vi "UNITEST MAIN.vi"() -> ()   [LabVIEW 2025]
uses:
  controls/LAB-IQ UI Data.ctl
  support/Message Queue/Enqueue Message (Single).vi
  <vilib>/Utility/error.llb/Error Cluster From Error Code.vi
  <vilib>/ErrorRing/Error Ring.xnode
  support/Message Queue/LAB-IQ Message Queue.lvlib
  support/User Event - Stop/LAB-IQ User Event - Stop.lvlib
panel:
  in  "Tab Control 3":T1(tab)
  in  "Tab Control 5":enum32{""}(tab)
  in  "Tab Control 14":T2(tab)=enum."Motor Load"
  out "sample temp":dbl caption="Sample Temperature" min=-200.0 max=200.0 step=0.1 format="%.1f"
  in  "output range":cluster{"output high":dbl, "output low":dbl}={"output high"=80.0, "output low"=0.0} {"output low" format="%.2f"; "output high" format="%.2f"}
  in  "PID gains out":T3={"proportional gain (Kc)"=40.0, "integral time (Ti, min)"=0.09, "derivative time (Td, min)"=0.0} {"derivative time (Td, min)" format="%.3f"; "integral time (Ti, min)" format="%.3f"; "proportional gain (Kc)" format="%.3f"}
  out "HT PID o/p":dbl
  in  "reinit":bool=TRUE
  out "gFF Rot 6":cluster{dbl, dbl, dbl}(graph)
  out "HT PID o/p 2":dbl
  in  "reinit 2":bool=TRUE
  in  "PID gains out 2":T3={"proportional gain (Kc)"=10.0, "integral time (Ti, min)"=1.667, "derivative time (Td, min)"=0.0} {"derivative time (Td, min)" format="%.3f"; "integral time (Ti, min)" format="%.3f"; "proportional gain (Kc)" format="%.3f"}
  in  "output range 3":cluster{"output high":dbl, "output low":dbl}={"output high"=80.0, "output low"=0.0} {"output low" format="%.2f"; "output high" format="%.2f"}
  out "gFF Rot 8":cluster{dbl, dbl, dbl}(graph)
  in  "Ramp MulFac":dbl=2.0
  in  "pulses LoadDiffRamp(2..10)":dbl=9.0
  in  "PulseControlRamp(diff<=3N)":dbl=5.0 min=1.0 max=1000.0 step=1.0 format="%#.1f"
  in  "SetLoadDeadband(%) Load(0-10N)":dbl=0.1 min=0.0001 max=100.0 step=0.0001 format="%#.6f"
  in  "PID gains out delay (microForce)":T3={"proportional gain (Kc)"=300.0, "integral time (Ti, min)"=0.00011, "derivative time (Td, min)"=0.0} {"derivative time (Td, min)" format="%.3f"; "integral time (Ti, min)" min=1e-05 max=100.0 step=1e-06 format="%.6f"; "proportional gain (Kc)" format="%.3f"}
  in  "Ramp":bool
  in  "Gain 2":dbl=0.016
  in  "pulses LoadDiff(2..10)":dbl=10.0
  in  "pulses LoadDiff(11..50)":dbl=40.0
  in  "PulseControl(diff<=3N)":dbl=1.0 min=1.0 max=1000.0 step=1.0 format="%#.1f"
  out "SetLoadDeadband(%)  2":dbl=1.0 min=0.001 max=100.0 step=0.001 format="%#.6f"
  in  "Dummy Run":bool
  out "Vertical load (N)":dbl format="%#.3f"
  in  "AutoTune":bool
  in  "Offset  3":dbl=1.5
  in  "apply load":bool
  in  "Enter ByPass Load":dbl
  in  "reinit 3":bool=TRUE
  in  "output range delay":cluster{"output high":dbl, "output low":dbl}={"output high"=100.0, "output low"=-100.0} {"output low" format="%.2f"; "output high" format="%.2f"}
  in  "PID gains out delay":T3={"proportional gain (Kc)"=30.0, "integral time (Ti, min)"=0.00101, "derivative time (Td, min)"=0.0} {"derivative time (Td, min)" format="%.3f"; "integral time (Ti, min)" min=1e-05 max=100.0 step=0.0001 format="%.4f"; "proportional gain (Kc)" format="%.3f"}
  in  "Bypass Load":bool
  in  "pulsesSent":dbl=200.0
  out "pulses":dbl
  out "actpid":dbl
  out "gFF Rot 7":cluster{dbl, dbl, dbl}(graph)
  in  "pulses LoadDiff(21..1000)":dbl=40.0
  in  "Delay":dbl=1.5 min=0.001 max=5.0 step=0.001 format="%#.6f"
  in  "deadband":dbl=0.2
  in  "Tab Control 26":enum32{"Page 1", "Page 2"}(tab)
  in  "ClearAll":bool
  out "Mz(Nm)":dbl[](array[numeric])
  out "My(Nm)":dbl[](array[numeric])
  out "Mx(Nm)":dbl[](array[numeric])
  in  "Save Dwell":dbl=0.015 caption="Save Dwell (sec)" min=0.0 max=5.0 step=0.001 format="%.3f"
  out "Set Speed 2":dbl
  out "Mx":dbl[](graph)
  out "My":dbl[](graph)
  out "Mz":dbl[](graph)
  out "Fx(N)":dbl[](graph)
  out "Fy(N)":dbl[](graph)
  out "Fz(N)":dbl[](graph)
  in  "ZeroAll":bool
  in  "Acq Delay (ms)":dbl=10.0
  in  "Burst Delay (ms)":dbl=10.0
  out "model":string
  out "SN":i32
  out "FFx(N)":dbl[](array[numeric])
  in  "Sensor IP":string="192.168.1.100"
  in  "Port":i32=8080
  out "FFy(N)":dbl[](array[numeric])
  out "Load(N)":dbl[](array[numeric])
  out "AE":bool
  in  "delete Handle":bool
  in  "Create Handle":bool=TRUE
  out "ft_data":dbl[](array[numeric])=[1.0, 1.0, 1.0, 1.0, 1.0, 1.0]
  out "ft_range":dbl[](array[numeric])=[1.0, 1.0, 1.0, 1.0, 1.0, 1.0]
  in  "stop 6":bool
  out "running_flag":bool
  out "ft_udp_handle":i32
  out "get-data-return":i32
  out "get-range-return":i32
  out "zero-return":i32
  out "filter-return":i32
  out "initial-return":i32
  out "deleteHandle-result":i32
  out "NL Kg":dbl caption="Normal Kg" min=-2000.0 max=2000.0 step=1.0 format="%.2f"
  in  "zFF 4":bool
  in  "APPLY":bool
  in  "Bypass":bool caption="Bypass to Manual load"
  in  "SP":dbl caption="SV ( N )" min=0.0 max=550.0 step=0.1 format="%.1f"
  in  "EGUpM":dbl=1500.0
  in  "Bypass 3":bool caption="Bypass  PID"
  in  "Control voltage":dbl caption="Control Voltage" min=0.0 max=10.0 step=0.01 format="%#.3f"
  out "NL":dbl caption="Normal Load ( N )" min=-2000.0 max=2000.0 step=1.0 format="%.2f"
  in  "Load 3":bool
  in  "Timer":dbl=1.0 min=0.0 max=50.0 step=1.0 format="%#.0f"
  out "Slide":dbl(slide) min=0.0 max=5.0 step=0.0001 scale=0.0..9.18
  in  "Approach \nVoltage":dbl min=0.0 max=2.0 step=0.01 format="%.2f"
  in  "PID gains < 10":T3={"proportional gain (Kc)"=0.032999999999999995, "integral time (Ti, min)"=0.019000000000000003, "derivative time (Td, min)"=0.0}
  in  "output range 2":cluster{"output high":dbl, "output low":dbl}={"output high"=9.18, "output low"=0.0}
  out "Chart 9":T4(graph)
  out "step size":i32=1
  out "Set Time":dbl
  out "Load 2":dbl
  out "Step Timer":dbl format="%<%H:%M:%S>t"
  in  "Sequence Counter":dbl
  in  "No of Sequence":i32 min=0 max=450 step=1
  in  "Depth gain R":dbl=0.5
  in  "Depth gain L":dbl=0.005
  out "Depth 2":cluster{dbl, dbl}(graph)
  out "HT PID output 2":dbl(slide) scale=0.0..100.0
  in  "zFF 5":bool
  out "FrictionKg":dbl caption="Friction Kg" min=-2000.0 max=2000.0 step=1.0 format="%.2f"
  out "friction":dbl caption="friction N" min=-2000.0 max=2000.0 step=1.0 format="%.2f"
  out "XY Graph 23":cluster{"scratch array-x":dbl[], dbl[]}(graph)
  out "XY Graph 24":cluster{"scratch array-x":dbl[], dbl[]}(graph)
  out "XY Graph 14":cluster{"scratch array-x":dbl[], dbl[]}(graph)
  out "XY Graph 13":cluster{"scratch array-x":dbl[], dbl[]}(graph)
  out "XY Graph 12":cluster{"scratch array-x":dbl[], dbl[]}(graph)
  in  "Tab Control 19":enum32{"Platform COM", "Config ", "DevInfo"}(tab)=enum."Config "
  in  "SAMPLES":dbl=100.0
  in  "Re-initilaize":bool
  in  "Filter ON/OFF":bool=TRUE
  in  "TracHomeSurgeOffsetCounts 10MM":dbl=505100.0
  in  "TracHomeSwayOffsetCounts 10MM":dbl=1432.0
  in  "Acoustic Emission:":dbl=1.0 min=0.0001 max=200.0 step=0.0001 format="%.4f"
  in  "Apply Filter (FF)":bool
  in  "Filter% 2":dbl=50.0 min=50.0 max=100.0 step=0.1 format="%.1f"
  in  "Apply Filter (Load)":bool=TRUE
  in  "Filter%":dbl=80.0 min=50.0 max=100.0 step=0.1 format="%.1f"
  in  "Sway distance (mm)":dbl=245.0
  in  "Surge distance (mm)":dbl=370.0
  in  "DataSavingLoopDelay(ms)":dbl=15.0
  in  "SAVE  2":bool
  in  "Enter Distance":bool caption="Enter Counts"
  in  "Sway Counts:":dbl=100.0 min=0.0 max=100000000.0 step=1.0 format="%.2f"
  in  "Distance (mm): 3":dbl=100.0 caption="Distance (mm):" min=0.0 max=1500.0 step=0.001 format="%.5f"
  in  "Surge Counts:":dbl=100.0 min=0.0 max=100000000.0 step=1.0 format="%.1f"
  in  "Distance (mm): 2":dbl=100.0 caption="Distance (mm):" min=0.0 max=1500.0 step=0.0001 format="%.3f"
  in  "Distance (mm):":dbl=100.0 min=0.0 max=1500.0 step=0.001 format="%.5f"
  in  "Heave Counts:":dbl=100.0 min=0.0 max=100000000.0 step=1.0
  in  "LRMHomeSurgeOffsetCounts":dbl=307197.0
  in  "LRMHomeSwayOffsetCounts":dbl=26880.0
  in  "TracHomeSurgeOffsetCounts 20MM":dbl=505100.0
  in  "TracHomeSwayOffsetCounts 20MM":dbl=1432.0
  in  "RotHomeSwayOffsetCounts":dbl=14656.0
  in  "RotHomeSurgeOffsetCounts":dbl=311465.0
  in  "Heave distance":dbl=340.0
  out "Zmm":dbl=1600.0
  out "Heave Pulses/mm":dbl=1600.0
  out "Surge Pulses/mm":dbl=1600.0
  out "Sway Pulses/mm":dbl=320.0
  in  "Heave Pitch":dbl=4.0
  in  "Surge Pitch":dbl=3.0
  in  "Sway Pitch":dbl=2.0
  in  "Heave PPR":dbl=6400.0
  in  "Surge PPR":dbl=6400.0
  in  "Sway PPR":dbl=6400.0
  in  "Step Speed":enum32{"Step Speed", "Step (load-Speed)"}(tab)
  in  "StepTable For Speed":string[][](table)=[["", "", ""], ["", "", ""], ["", "", ""], ["", "", ""]]
  in  "StepTable For Load-Speed":string[][](table)=[["", "", ""], ["", "", ""], ["", "", ""], ["", "", ""]]
  in  "GUI":T5(tab)
  in  "Platform Settings":bool caption="Password"
  in  "Configure":bool caption="Password"
  in  "Home":bool caption="Password"
  in  "EXIT":bool
  in  "Analysis":bool caption="Password"
  in  "service 2":bool caption="Password"
  in  "MainPage":T6(tab)=enum."HOME"
  in  "Select Load Head":bool
  in  "Notes :":string
  in  "FILE":string
  in  "Sample ID :":string
  in  "Operator ID :":string
  in  "Operator Name :":string
  in  "Auto":bool caption="Power Status"
  out "mm/s  Surge":dbl=7.0 caption="Jog" min=0.001 max=50.0 step=0.0001 format="%.2f"
  in  "Update Surge Speed":bool
  out "Drive Error":string
  in  "Disable Axis Jog Soft Limits":bool
  out "mm/s  Sway":dbl=7.0 caption="Jog" min=0.001 max=50.0 step=0.0001 format="%.2f"
  out "Sway and Surge COM Status":bool=TRUE caption="Load COM Status"
  out "Heave COM Status":bool=TRUE caption="Load COM Status"
  in  "Enable Platform":bool
  in  "Surge Forward Main":bool
  in  "Surge Backward Main":bool
  in  "Sway Right Main":bool
  in  "Sway Left Main":bool
  in  "Heave Down Main":bool
  in  "Heave Up main":bool
  in  "Update Sway Speed":bool
  in  "Update Heave Speed":bool
  out "mm/s Heave":dbl=7.0 caption="Jog" min=0.001 max=30.0 step=0.0001 format="%.2f"
  in  "mm/sec":dbl=1.0 caption="Jog" min=0.001 max=50.0 step=0.001 format="%.2f"
  in  "mm":dbl=0.001 caption="Jog" min=0.001 max=200.0 step=0.0001 format="%#.3f"
  in  "Surface Analysis":bool
  in  "Imaging":bool
  in  "Image Analysis":bool
  in  "Post Analysis":bool
  in  "Enter the Loading Rate (N/min)":dbl=60.0 min=60.0 max=1200.0 step=0.1 format="%.2f"
  out "Message":string="Load Entered is out of range!!!"
  out "Warning 2":bool
  in  "SSP 0.75":bool
  in  "SSP 0.5":bool
  in  "SSP 0.3":bool
  in  "Warning":enum32{"Page 2"}(tab)
  in  "gui GIF":enum32{"Check", "Deca", "kilo", "Micro"}(tab)
  out "Communication is established":bool=TRUE caption="Load COM Status"
  in  "AppLoad 4":bool
  in  "Multipoint":bool caption="Singlepoint"
  in  "Indentation":string[][](table)=[["Detection", "5", "2"], ["Unload", "0", "5"], ["Load", "10", "2"], ["Unload", "0", "5"], ["Detection", "5", "2"], ["Unload", "0", "5"]]
  in  "Reference Sample":u16(ring) items=["None", "Brass", "Aluminium", "Mild Steel"]
  out "Load Cell Communication Slide":u8(slide)=1 min=1 max=10 step=1 scale=0.0..10.0
  in  "com 3":bool
  out "com":bool
  out "DecaForce COM Status":bool caption="Load COM Status"
  in  "Update":bool
  in  "Clear 3":bool
  in  "seq":bool=TRUE
  in  "Stribeck table":bool
  in  "Stribeck Table  For loading":string[][](table)=[["", "", ""], ["", "", ""], ["", "", ""], ["", "", ""]]
  in  "Loading Mode":u16(ring) items=["Constant", "Ramp", "Steps", "Indentation"]
  in  "Enter the Final Load (N)":dbl=1.0 min=0.0 max=500.0 step=1.0 format="%#.0f"
  in  "Enter the CoF Trip":dbl=1.0
  in  "Enter the Friction Force Trip":dbl=520.0 min=500.0 max=500.0 step=1.0 format="%#.1f"
  in  "Enter the Normal load Trip":dbl=520.0 min=500.0 max=500.0 step=0.001 format="%.3f"
  in  "Enter the Load  (N)":dbl=2.0 min=0.0 max=500.0 step=0.1 format="%#.4f"
  in  "KiloForce":bool
  in  "DecaForce":bool
  in  "MicroForce":bool
  in  "LHBack":bool
  in  "LHNext":bool
  in  "zNL":bool
  out "NL disp":dbl caption="Normal Load ( N )" min=-2000.0 max=2000.0 step=0.0001 format="%.1f"
  in  "Rotary Tab":enum32{"Page 1", "Page 2"}(tab)
  in  "Motion Direction:  3":u16(ring) items=["Clockwise", "Counter Clockwise"]
  in  "E.Velocity 2":bool=TRUE caption="SRR"
  out "e.v/ssr 2":enum32{"E.V", "SSR"}(tab)
  in  "Enter Fixed SRR 2":dbl min=0.0 max=0.0 format="%.3f"
  in  "Enter the Final E.Velocity (m/s) 2":dbl=1.0 min=0.001 max=4.0 step=0.001 format="%.3f"
  in  "Enter initial E.Velocity (m/s) 2":dbl=2.0 min=0.001 max=4.0 step=0.001 format="%.3f"
  in  "Enter Fixed E.Velocity 2":dbl=1.0 min=0.001 max=2.0 step=0.001 format="%.3f"
  in  "Enter Final SRR 2":dbl=1.0 min=0.001 max=1.0 step=0.001 format="%.2f"
  in  "Enter initial SRR 2":dbl=1.0 min=0.001 max=1.0 step=0.001 format="%.2f"
  out "Final Speed (RPM) 3":dbl=1.0 min=0.1 max=3000.0 step=0.1 format="%.1f"
  out "Initial Speed (RPM) 2":dbl=100.0 min=0.1 max=3000.0 step=0.1 format="%.1f"
  in  "Enter the Final Velocity (m/s) 3":dbl=1.0 min=0.001 max=2.0 step=0.001 format="%.3f"
  in  "Enter initial Velocity (m/s)  3":dbl=2.0 min=0.001 max=2.0 step=0.001 format="%.3f"
  out "Ramp Up 2":bool caption="Ramp Down"
  in  "TEST SELECTION":enum32{"Time", "Cycle"}(radio)
  in  "SPEED SELECTION :":enum32{"Speed in RPM", "Speed in m/sec"}(radio)=enum."Speed in m/sec"
  in  "Angular Oscillation Set":bool
  in  "Traction":bool
  in  "Surge Forward MM":bool
  in  "Surge Backward MM":bool
  in  "M3 Image":enum32{"Page 1", "Page 2"}(tab)
  in  "String 39":string="Jog heave to bring the upper sample closer to the lower sample within 1mm."
  in  "Sway Left MM":bool
  in  "Sway Right MM":bool
  in  "Disable Axis Jog Soft Limits":bool
  in  "mm":dbl=0.001 caption="Jog" min=0.001 max=5.0 step=0.0001 format="%#.3f"
  in  "Heave Down MM":bool
  in  "Heave Up MM":bool
  in  "Wear Track Diameter (mm)":dbl=5.0 caption="Wear Track Diameter (mm):" min=1.0 max=30.0 step=1.0 format="%.2f"
  in  "Set WTD":bool
  in  "HomeScratch":bool
  in  "HomeRot":bool
  in  "PlaceModule":bool
  in  "Enter the Angle (Deg)":dbl=45.0 min=5.0 max=300.0 step=1.0
  in  "Enter the Frequency (Hz)":dbl=1.0 min=0.1 max=10.0 step=0.1 format="%.1f"
  in  "Motion Mode:":u16(ring) items=["Uniform Rotation", "Angular Oscillation", "Stribeck ", "Steps"]
  in  "LR Sway":bool
  in  "Rot Hor":bool
  in  "Rot Ver":bool
  in  "Scratch":bool
  in  "LR Cam":bool
  in  "MMBack":bool
  in  "MMNext":bool
  out "Humidity  Status  3":bool caption="Communication Status"
  out "Low Temp  Status  2":bool caption="Communication Status"
  out "TK4 status 2":bool caption="Communication Status"
  in  "String 40":string="Before selecting Acoustic make sure the sensor output pin is connected to A4."
  in  "Stage Temperature":dbl[](array[numeric])=[150.0, 230.0, 300.0, 350.0, 400.0, 450.0, 500.0]
  in  "Sample Temperature":dbl[](array[numeric])=[100.0, 150.0, 200.0, 250.0, 300.0, 350.0, 400.0]
  in  "Humidity (Amb)":bool
  in  "Clear List":bool
  out "Sensors Picked":string
  in  "Add to list":bool
  in  "Wear":bool
  in  "Vibration":bool
  in  "Humidity (Chamber)":bool
  in  "Temperature (Chamber)":bool
  in  "ECR":bool
  in  "Temperature (Amb)":bool
  in  "Microphone":bool
  in  "Acoustic Emission 3":bool
  in  "SNext":bool
  in  "APBack":bool
  in  "Enter the Temperature (°C):":dbl
  in  "Enter the Stage \nTemperature (°C):":dbl=20.0 min=20.0 max=150.0 step=1.0 format="%#.0f"
  in  "Enter the Humidity (%Rh):":dbl=30.0 min=30.0 max=85.0 step=1.0
  in  "Low Temp":bool
  in  "High Temp":bool
  in  "Humidity":bool
  in  "Main Screen Tab":T7(tab)
  in  "AppLoadSeq scratch":bool
  in  "Stop Scratch":bool
  in  "ClrLog":bool
  out "Trip Log":string
  in  "STOP":bool
  in  "Start Test":bool
  out "Test status":bool caption="Test Status"
  out "AR Led":bool caption="AR"
  out "Data":bool=TRUE
  out "Health":bool=TRUE
  out "Sway COM Status":bool=TRUE caption="Load COM Status"
  out "Heave COM Status":bool=TRUE caption="Load COM Status"
  in  "Grp Tab":enum32{"Rot/LRM", "FBT"}(tab)
  in  "Sub Graph":T8(tab)
  in  "Speed Reset Graph":bool
  in  "Speed Tab":enum32{" Rotary Disc", "MTM Ball", "MTM Disc"}(tab)
  out "speed mm/sec":dbl(graph)=0.13298760003255525
  out "MTM BALL SPEED":dbl(graph)=0.13298760003255525
  out "MTM DISC  SPEED":dbl(graph)=0.13298760003255525
  in  "Temperature Reset":bool
  out "Temperature (deg c)":dbl(graph)=0.13298760003255525
  in  "ECR RESET":bool
  out "ECR":dbl(graph)=0.13298760003255525
  out "Acoustic Emission (mV)":dbl min=0.0 max=5000.0 step=0.1
  in  "Aqucostic Reset Graph":bool
  out "gACQUOS":dbl(graph)=0.13298760003255525
  in  "Humidity Reset Graph":bool
  out "HumrGp":dbl(graph)=0.13298760003255525
  out "SD (mm)":dbl caption="Sliding Distance ( mm )" min=-200.0 max=200.0 step=0.1 format="%.4f"
  in  "Siliding distance Reset Graph":bool
  out "SDGp":dbl(graph)=0.13298760003255525
  out "Hymidity":bool
  in  "Humidity Disable trip":bool=TRUE
  in  "CoF Trip  2":dbl=540.0 min=100.0 max=540.0 step=1.0
  out "Depth Trip":dbl=600.0
  in  "Depth Trip":bool=TRUE
  out "Weart Deapth":bool
  in  "Depth Reset Graph":bool
  out "Weart":bool
  in  "Depthz":bool
  out "Depth (µm)":dbl min=-200.0 max=200.0 step=0.1 format="%.1f"
  out "WearGp":dbl(graph)=0.13298760003255525
  out "NL Trip 2":dbl=600.0
  out "Load pid":bool
  in  "Load Disable Trip":bool=TRUE
  in  "Load Reset Graph":bool
  out "NL Display 4":dbl caption="Normal Load ( N )" min=-2000.0 max=2000.0 step=0.0001 format="%.1f"
  out "Main Chart 3":cluster{dbl, "NL disp":dbl, dbl}(graph)
  in  "BACK":bool
  out "Ambient \nTemperature":dbl min=0.0 max=5000.0 step=0.1 format="%.1f"
  out "Ambient\n Humidity":dbl min=0.0 max=5000.0 step=0.1 format="%.2f"
  out "NL disp 2":dbl caption="Normal Load ( N )" min=-2000.0 max=2000.0 step=0.0001 format="%.1f"
  out "Set Humidity":dbl caption="Set Humidity  (% Rh)" min=-2000.0 max=2000.0 step=1.0 format="%.1f"
  out "humidity disp":dbl caption="Humidity (% Rh)" min=-2000.0 max=2000.0 step=1.0 format="%.1f"
  in  "Humidity On":bool
  in  "zNL 2":bool
  out "NLt":bool
  in  "Load En":bool
  out "Freq (Hz)":dbl min=0.0 max=5000.0 step=0.1 format="%.4f"
  out "HumCOMStatus":bool caption="Communication Status"
  out "Load Communication":bool
  in  "Temp Tabs":enum32{"Low Temp", "High Temp"}(tab)
  out "Controller  Status":bool
  out "ChamberTemp":dbl format="%#.1f"
  in  "SetTmp":dbl=-190.0 caption="Set Temperature (Deg C)" min=-190.0 max=100.0 step=1.0 format="%.1f"
  in  "Cooling":bool
  in  "Heater":bool
  out "TK4 status":bool caption="Controller  Status"
  out "ChamberTemp":dbl format="%#.1f"
  in  "SetTmp":dbl caption="Set Temperature (Deg C)" min=0.0 max=1000.0 step=1.0 format="%.1f"
  in  "Set Load (N)":dbl=100.0 min=0.01 max=1500.0 step=0.01 format="%.1f"
  in  "Time Tab":enum32{"cycles", "duration"}(tab)
  out "Test Duration 4":dbl=600.0 caption="Test Duration\n(HH:MM:SS)" min=0.0083 max=180000.0 step=0.0001 format="%<%H:%M:%S>t"
  out "TEST CYCLE":dbl min=0.0 max=5000.0 step=0.01 format="%.2f"
  in  "TOTAL CYCLES":dbl min=0.0 max=5000.0 step=0.1 format="%.4f"
  out "Time ( HH:MM:SS ) 2":dbl min=0.0 max=144000.0 step=1.0 format="%<%H:%M:%S>t"
  in  "Test Duration":dbl=600.0 caption="Test Duration\n(HH:MM:SS)" min=0.0083 max=180000.0 step=0.0001 format="%<%H:%M:%S>t"
  in  "Main Speed Tab":enum32{"ROTARY", "TRACTION"}(tab)
  in  "SPEED TAB":enum32{"RPM", "m/sec"}(tab)
  out "Speed (RPM)":dbl min=0.0 max=5000.0 step=0.1 format="%.1f"
  out "Set Speed":dbl caption="Set Speed (RPM)" min=0.0 max=1500.0 step=0.1 format="%.1f"
  out "Speed (m/sec)":dbl min=0.0 max=5000.0 step=0.001 format="%.4f"
  out "Set Speed (m/sec)":dbl min=0.0 max=1500.0 step=0.001 format="%.4f"
  in  "MTM MOTOR DISPLAY":enum32{"MTM RPM", "MTM m/sec"}(tab)
  out "Disc Speed (RPM)":dbl min=0.0 max=1500.0 step=0.1 format="%.1f"
  out "Ball Speed (RPM)":dbl min=0.0 max=1500.0 step=0.1 format="%.1f"
  out "Disc Speed (m/sec)":dbl min=0.0 max=1500.0 step=0.1 format="%.1f"
  out "Ball Speed (m/sec)":dbl min=0.0 max=1500.0 step=0.1 format="%.1f"
  in  "Angle and Frequency":enum32{"angular", "lrm"}(tab)
  out "Angle (Deg)":dbl min=0.0 max=5000.0 step=0.01 format="%.2f"
  out "Stroke (mm)":dbl min=0.0 max=5000.0 step=0.01 format="%.2f"
  in  "Analysis Home":bool
  in  "Password":string
  in  "Home Service":bool
  in  "Advanced Setting":bool
  in  "About Tab":enum32{"Primary"}(tab)
  in  "ECR Port:":refnum<visa-resource-name>="COM10"
  in  "Ramp Port:":refnum<visa-resource-name>="COM10"
  in  "Installation/Replacement completed":bool
  in  "Loahead":bool
  in  "Heave and Surge COM Port:":refnum<visa-resource-name>="COM9"
  in  "Sway COM Port:":refnum<visa-resource-name>="COM10"
  in  "Temp Modbus:":refnum<visa-resource-name>="COM14"
  in  "Humidity Port:":refnum<visa-resource-name>="COM10"
  in  "Edit Gain Constants":bool
  in  "Save Gain Constants":bool
  in  "Service About":bool
  # "load Aquisition off"
  # "load Aquisition On"
  # "Configuration"
  # "Limits for Heave Surge and Sway"
  # "Modules Offset Parameters"
  # "Counts-Distance Calculator"
  # "File Name :"
  # "Ensure the traction module is aligned\n horizontally with the stage before ENABLE."
  # "SET JOG SPEED"
  # "JOG MODE"
  # "Module Selection"
  # "Positioning Control"
  # "Connect the controller\ncable to M3"
  # "Environment"
  # "Sensors"
  # "Data Points"
  # "Data Points"
  # "Data Points"
  # "Data Points"
  # "ohms"
  # "Data Points"
  # "Data Points"
  # "Data Points"
  # "LAB-IQ 150 / UNITEST / WO2456 / UT150  v05 / AUGUST 2025"
  # "NOTE: This operation needs to be done only when the machine is ON."
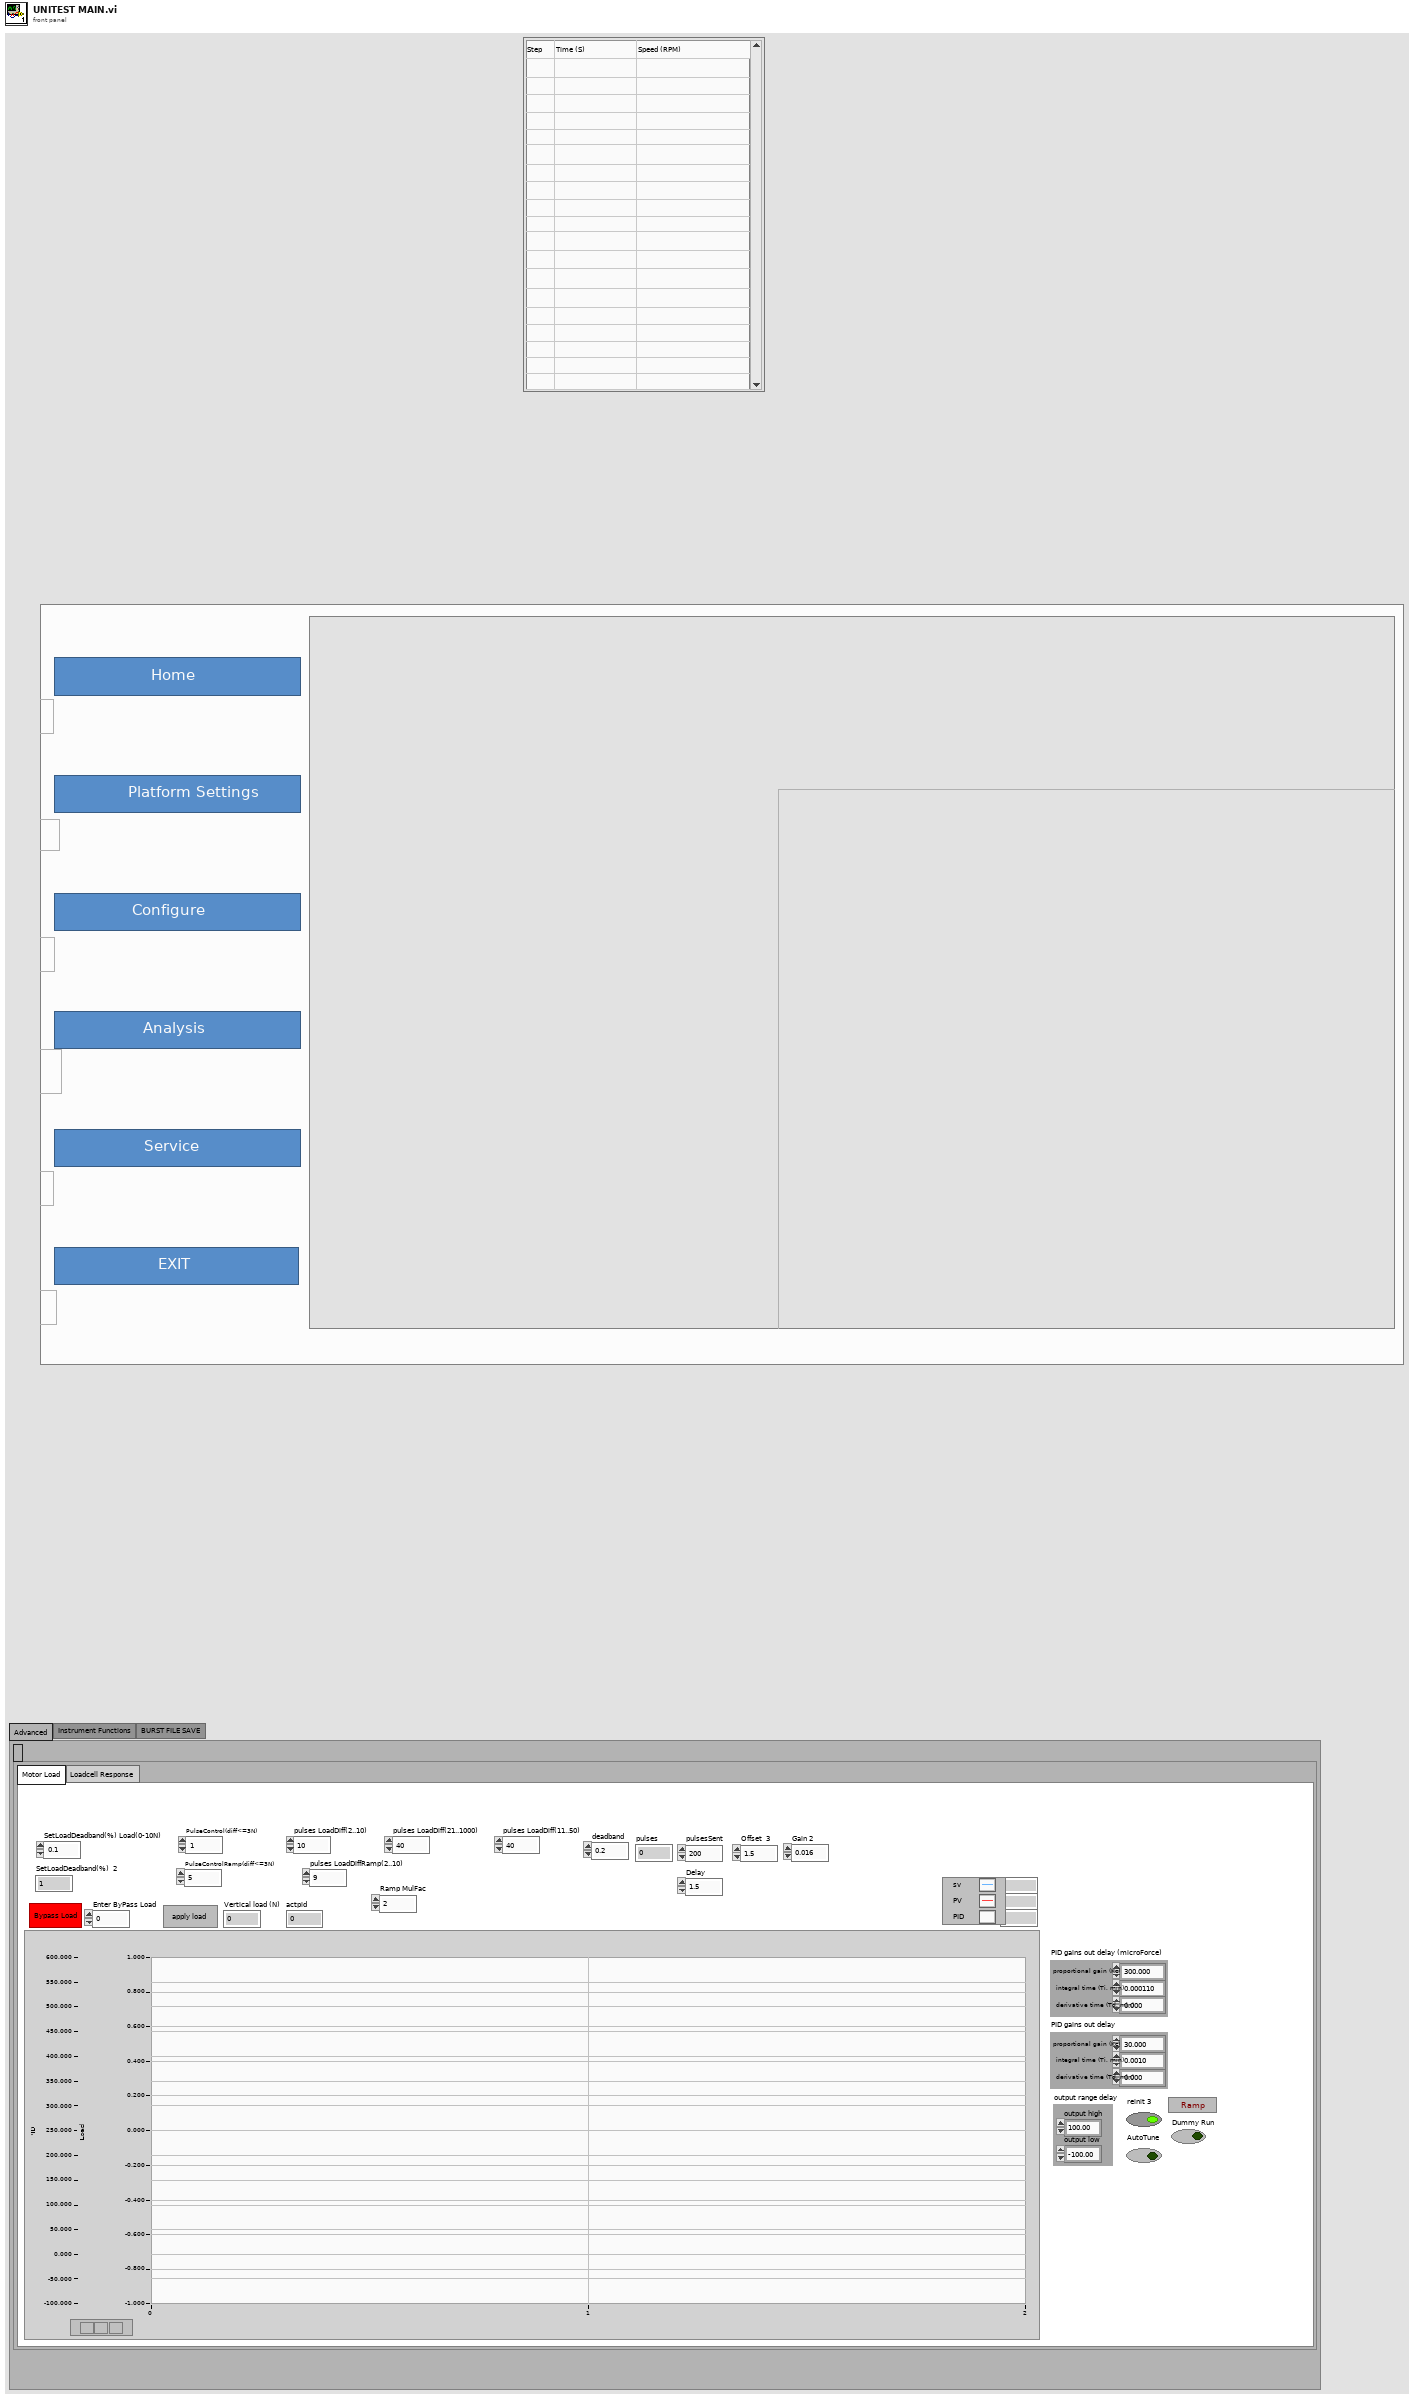
[diagram p1: front panel]
types:
  T1 = enum32{"Advanced", "Motor", "Depth_graph", "UIO Communicator", "Add to list parametrs", "Instrument Functions", "BURST FILE SAVE"}
  T2 = enum32{"LRM heating", "FBT_Heating", "Motor Load", "Loadcell Response", "Voice Load", "Step loading and speed ", "Depth"}
  T3 = cluster{"proportional gain (Kc)":dbl, "integral time (Ti, min)":dbl, "derivative time (Td, min)":dbl}
  T4 = cluster{dbl, "NL ONLINE ( N )":dbl, "output":dbl}
  T5 = enum32{"Setup", "Load Head", "Motion Module", "Environment", "Begin"}
  T6 = enum32{"Details", "PlatformSetting", "Analysis", "HOME"}
  T7 = enum32{"  Acquire  ", "Compare Files Rot", "About", "Service"}
  T8 = enum32{"Speed", "Temperature", "ECR", "Acoustic Emission", "Humidity", "Sliding Distance"}
  T9 = typedef "LAB-IQ UI Data.ctl" = cluster{"Main Home Screen":cluster{"GUI":refnum<vi>, "Platform Settings":refnum<vi>, "Configure":refnum<vi>, "Home":refnum<vi>, "EXIT":refnum<vi>, "service 2":refnum<vi>, "MainPage":refnum<vi>, "Analysis":refnum<vi>}, "Platform Settings":cluster{"mm/s  Surge":refnum<vi>, "Update Surge Speed":refnum<vi>, "Drive Error":refnum<vi>, "Disable Axis Jog Soft Limits":refnum<vi>, "mm/s  Sway":refnum<vi>, "Sway and Surge COM Status":refnum<vi>, "Heave COM Status":refnum<vi>, "Enable Platform":refnum<vi>, "Surge Forward Main":refnum<vi>, "Sway Right Main":refnum<vi>, "Sway Left Main":refnum<vi>, "Heave Down Main":refnum<vi>, "Heave Up main":refnum<vi>, "Update Sway Speed":refnum<vi>, "Update Heave Speed":refnum<vi>, "mm/s Heave":refnum<vi>, "mm/sec":refnum<vi>, "mm":refnum<vi>, "Surge Backward Main":refnum<vi>}, "Analysis Screen":cluster{"Analysis Home":refnum<vi>, "Surface Analysis":refnum<vi>, "Imaging":refnum<vi>, "Image Analysis":refnum<vi>, "Post Analysis":refnum<vi>}, "Config Screen":cluster{"Select Load Head":refnum<vi>, "Notes :":refnum<vi>, "FILE":refnum<vi>, "Sample ID :":refnum<vi>, "Operator ID :":refnum<vi>, "Operator Name :":refnum<vi>, "Auto":refnum<vi>}, "Motion Module":cluster{"zNL":refnum<vi>, "NL disp":refnum<vi>, "Rotary Tab":refnum<vi>, "Motion Direction:  3":refnum<vi>, "E.Velocity 2":refnum<vi>, "e.v/ssr 2":refnum<vi>, "Enter Fixed E.Velocity 2":refnum<vi>, "Enter Final SRR 2":refnum<vi>, "Enter initial SRR 2":refnum<vi>, "Enter Fixed SRR 2":refnum<vi>, "Enter the Final E.Velocity (m/s) 2":refnum<vi>, "Enter initial E.Velocity (m/s) 2":refnum<vi>, "Final Speed (RPM) 3":refnum<vi>, "Initial Speed (RPM) 2":refnum<vi>, "Enter the Final Velocity (m/s) 3":refnum<vi>, "Enter initial Velocity (m/s)  3":refnum<vi>, "Ramp Up 2":refnum<vi>, "TEST SELECTION":refnum<vi>, "SPEED SELECTION : ":refnum<vi>, "Angular Oscillation Set":refnum<vi>, "Traction":refnum<vi>, "Step Speed":refnum<vi>, "StepTable For Load-Speed":refnum<vi>, "StepTable For Speed":refnum<vi>, "Surge Forward MM":refnum<vi>, "Surge Backward MM":refnum<vi>, "M3 Image":refnum<vi>, "String 39":refnum<vi>, "Sway Left MM":refnum<vi>, "Sway Right MM":refnum<vi>, "Disable Axis Jog Soft Limits":refnum<vi>, "mm":refnum<vi>, "Heave Down MM":refnum<vi>, "Heave Up MM":refnum<vi>, "Wear Track Diameter (mm)":refnum<vi>, "Set WTD":refnum<vi>, "HomeScratch":refnum<vi>, "HomeRot":refnum<vi>, "PlaceModule":refnum<vi>, "Enter the Angle (Deg)":refnum<vi>, "Enter the Frequency (Hz)":refnum<vi>, "Motion Mode:":refnum<vi>, "LR Sway":refnum<vi>, "Rot Hor":refnum<vi>, "Scratch":refnum<vi>, "LR Cam":refnum<vi>, "MMBack":refnum<vi>, "MMNext":refnum<vi>, "Rot Ver":refnum<vi>}, "Environmental control":cluster{"Humidity  Status  3":refnum<vi>, "Low Temp  Status  2":refnum<vi>, "TK4 status 2":refnum<vi>, "Stage Temperature":refnum<vi>, "Sample Temperature":refnum<vi>, "Humidity (Amb)":refnum<vi>, "Clear List":refnum<vi>, "Add to list":refnum<vi>, "Wear":refnum<vi>, "Vibration":refnum<vi>, "Humidity (Chamber)":refnum<vi>, "Temperature (Chamber)":refnum<vi>, "ECR ":refnum<vi>, "Temperature (Amb)":refnum<vi>, "Microphone":refnum<vi>, "Acoustic Emission 3":refnum<vi>, "SNext":refnum<vi>, "APBack":refnum<vi>, "Enter the Temperature (°C):":refnum<vi>, "Enter the Stage \nTemperature (°C):":refnum<vi>, "Enter the Humidity (%Rh):":refnum<vi>, "Low Temp":refnum<vi>, "High Temp":refnum<vi>, "Humidity":refnum<vi>, "Sensors Picked":refnum<vi>}, "About Screen":cluster{"Password":refnum<vi>, "Home Service":refnum<vi>, "Advanced Setting":refnum<vi>, "About Tab":refnum<vi>, "ECR Port:":refnum<vi>, "Ramp Port:":refnum<vi>, "Installation/Replacement completed":refnum<vi>, "Loahead":refnum<vi>, "Heave and Surge COM Port:":refnum<vi>, "Sway COM Port:":refnum<vi>, "Temp Modbus:":refnum<vi>, "Humidity Port:":refnum<vi>, "Edit Gain Constants":refnum<vi>, "Save Gain Constants":refnum<vi>}, "Main Screen":cluster{"Main Screen Tab":refnum<vi>, "Angle and Frequency":refnum<vi>, "Stroke (mm)":refnum<vi>, "Angle (Deg)":refnum<vi>, "Main Speed Tab":refnum<vi>, "MTM MOTOR DISPLAY":refnum<vi>, "Disc Speed (m/sec)":refnum<vi>, "Ball Speed (m/sec)":refnum<vi>, "Disc Speed (RPM)":refnum<vi>, "Ball Speed (RPM)":refnum<vi>, "SPEED TAB":refnum<vi>, "Speed (m/sec)":refnum<vi>, "Set Speed (m/sec)":refnum<vi>, "Speed (RPM)":refnum<vi>, "Set Speed":refnum<vi>, "Time Tab":refnum<vi>, "Time ( HH:MM:SS ) 2":refnum<vi>, "Test Duration":refnum<vi>, "Test Duration 4":refnum<vi>, "TEST CYCLE":refnum<vi>, "TOTAL CYCLES":refnum<vi>, "Set Load (N)":refnum<vi>, "Temp Tabs":refnum<vi>, "Heater":refnum<vi>, "TK4 status":refnum<vi>, "ChamberTemp":refnum<vi>, "SetTmp":refnum<vi>, "Controller  Status":refnum<vi>, "ChamberTemp 2":refnum<vi>, "SetTmp 2":refnum<vi>, "Controller  Status 2":refnum<vi>, "ChamberTemp 3":refnum<vi>, "SetTmp 3":refnum<vi>, "Cooling":refnum<vi>, "Load Communication":refnum<vi>, "Ambient \nTemperature":refnum<vi>, "HumCOMStatus":refnum<vi>, "Ambient\n Humidity":refnum<vi>, "Freq (Hz)":refnum<vi>, "Load En":refnum<vi>, "NLt":refnum<vi>, "zNL 2":refnum<vi>, "Humidity On":refnum<vi>, "humidity disp":refnum<vi>, "Set Humidity":refnum<vi>, "NL disp 2":refnum<vi>, "Humidity On 2":refnum<vi>, "humidity disp 2":refnum<vi>, "Set Humidity 2":refnum<vi>, "NL disp 3":refnum<vi>, "AppLoadSeq scratch":refnum<vi>, "Stop Scratch":refnum<vi>, "ClrLog":refnum<vi>, "Trip Log":refnum<vi>, "STOP":refnum<vi>, "Start Test":refnum<vi>, "Test status":refnum<vi>, "AR Led":refnum<vi>, "Data":refnum<vi>, "Health":refnum<vi>, "Sway COM Status":refnum<vi>, "Heave COM Status":refnum<vi>, "Grp Tab":refnum<vi>, "Sub Graph":refnum<vi>, "SD (mm)":refnum<vi>, "Siliding distance Reset Graph":refnum<vi>, "SDGp":refnum<vi>, "Humidity Reset Graph":refnum<vi>, "HumrGp":refnum<vi>, "Acoustic Emission (mV)":refnum<vi>, "Aqucostic Reset Graph":refnum<vi>, "gACQUOS":refnum<vi>, "ECR RESET":refnum<vi>, "ECR":refnum<vi>, "Temperature Reset":refnum<vi>, "Acoustic Emission (mV) 2":refnum<vi>, "Aqucostic Reset Graph 2":refnum<vi>, "gACQUOS 2":refnum<vi>, "ECR RESET 2":refnum<vi>, "ECR 2":refnum<vi>, "Temperature Reset 2":refnum<vi>, "Temperature (deg c)":refnum<vi>, "Speed Reset Graph":refnum<vi>, "Speed Tab":refnum<vi>, "MTM DISC  SPEED":refnum<vi>, "MTM BALL SPEED":refnum<vi>, "speed mm/sec":refnum<vi>, "Hymidity":refnum<vi>, "Humidity Disable trip":refnum<vi>, "CoF Trip  2":refnum<vi>, "Depth Trip":refnum<vi>, "Weart Deapth":refnum<vi>, "Depth Reset Graph":refnum<vi>, "Weart":refnum<vi>, "Depthz":refnum<vi>, "Depth (µm)":refnum<vi>, "WearGp":refnum<vi>, "NL Trip 2":refnum<vi>, "Load pid":refnum<vi>, "Load Disable Trip":refnum<vi>, "Load Reset Graph":refnum<vi>, "NL Display 4":refnum<vi>, "Main Chart 3":refnum<vi>, "BACK":refnum<vi>, "Depth Trip 2":refnum<vi>}, "Loading":cluster{"Indentation":refnum<vi>, "Reference Sample":refnum<vi>, "Load Cell Communication Slide":refnum<vi>, "com 3":refnum<vi>, "com":refnum<vi>, "DecaForce COM Status":refnum<vi>, "Update":refnum<vi>, "Clear 3":refnum<vi>, "seq":refnum<vi>, "Stribeck table":refnum<vi>, "Stribeck Table  For loading":refnum<vi>, "Loading Mode":refnum<vi>, "Enter the Final Load (N)":refnum<vi>, "Enter the CoF Trip":refnum<vi>, "Enter the Friction Force Trip":refnum<vi>, "Enter the Normal load Trip":refnum<vi>, "Enter the Load  (N)":refnum<vi>, "KiloForce":refnum<vi>, "DecaForce ":refnum<vi>, "MicroForce":refnum<vi>, "LHBack":refnum<vi>, "LHNext":refnum<vi>, "Enter the Loading Rate (N/min)":refnum<vi>, "Message":refnum<vi>, "Warning 2":refnum<vi>, "SSP 0.75":refnum<vi>, "SSP 0.5":refnum<vi>, "SSP 0.3":refnum<vi>, "Warning":refnum<vi>, "gui GIF":refnum<vi>, "Communication is established":refnum<vi>, "AppLoad 4":refnum<vi>, "Multipoint":refnum<vi>}}
  T10 = typedef "init queue out loop.ctl" = cluster{"UI Loop":refnum<queue>, "LOAD COM LOOP ":refnum<queue>, "SWAY MOTOR COM LOOP":refnum<queue>, "HEAVE MOTOR COM LOOP":refnum<queue>, "TEMPERATURE COM LOOP":refnum<queue>, "RAMP MOTOR COM LOOP":refnum<queue>, "ECR PORT":refnum<queue>, "HUMIDITY COM PORT":refnum<queue>, "PROGRAM LOOP":refnum<queue>, "MONITOR LOOP":refnum<queue>, "REPORT":refnum<queue>, "LOAD PID":refnum<queue>}
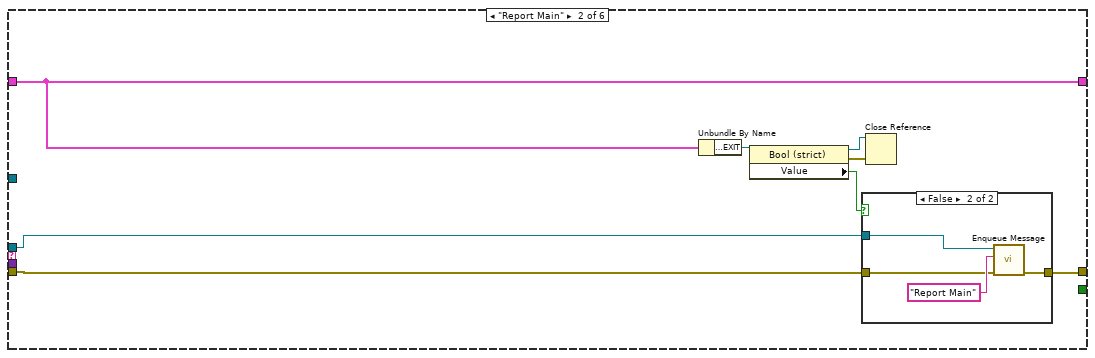
[diagram p2: hidden frame]
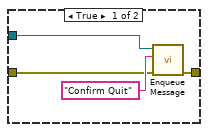
[diagram p3: hidden frame]
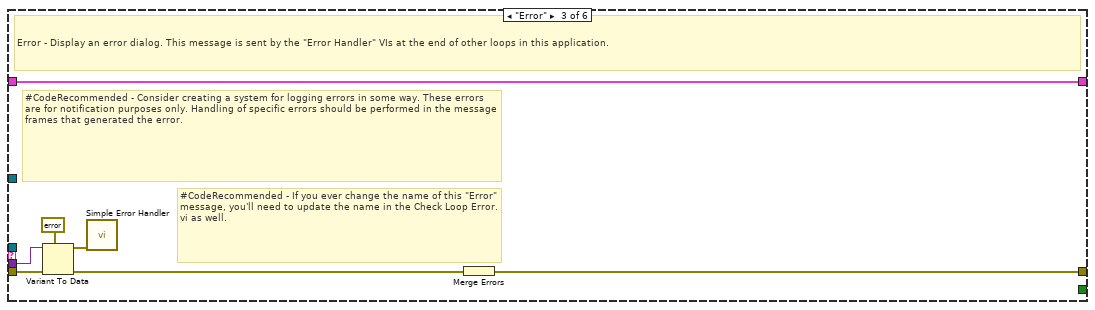
[diagram p4: hidden frame]
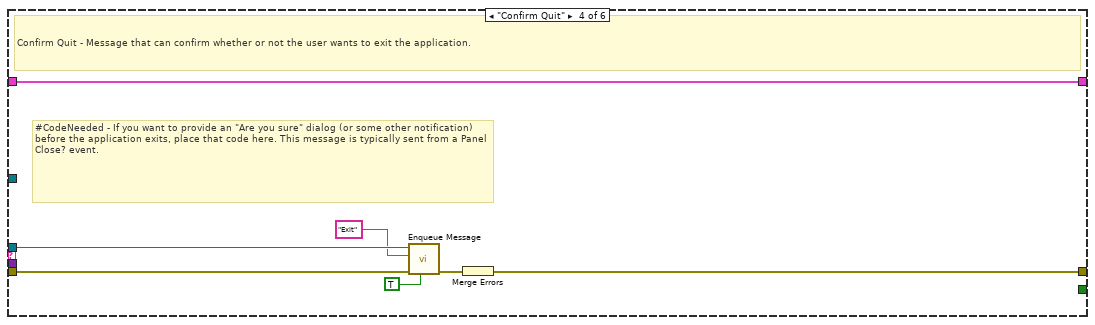
[diagram p5: hidden frame]
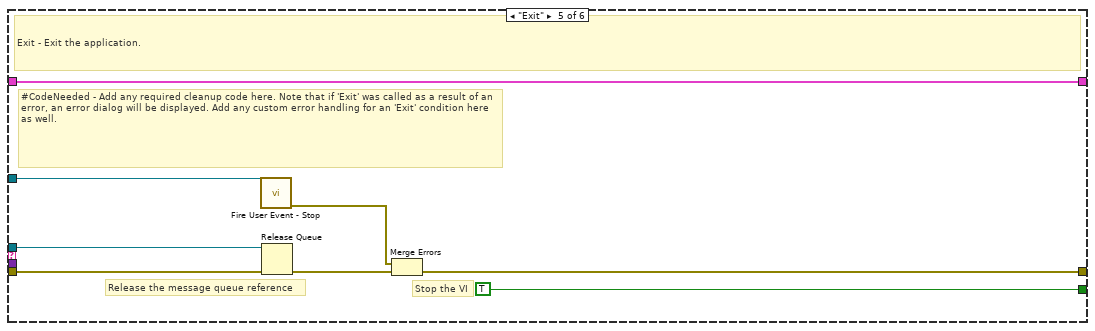
[diagram p6: hidden frame]
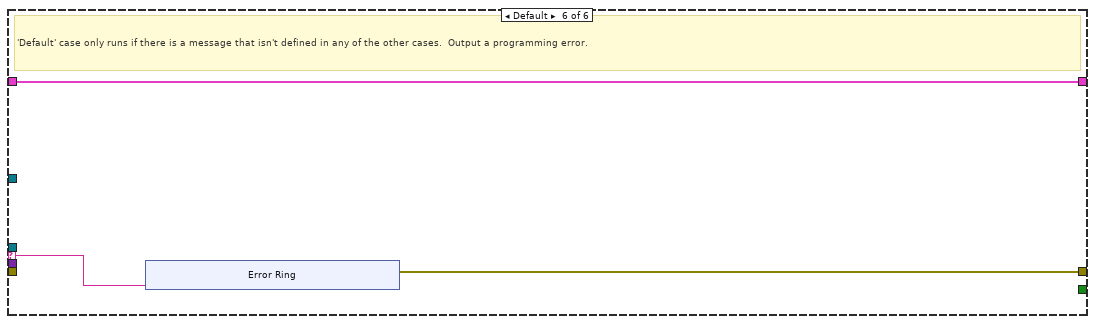
[diagram p7: hidden frame]
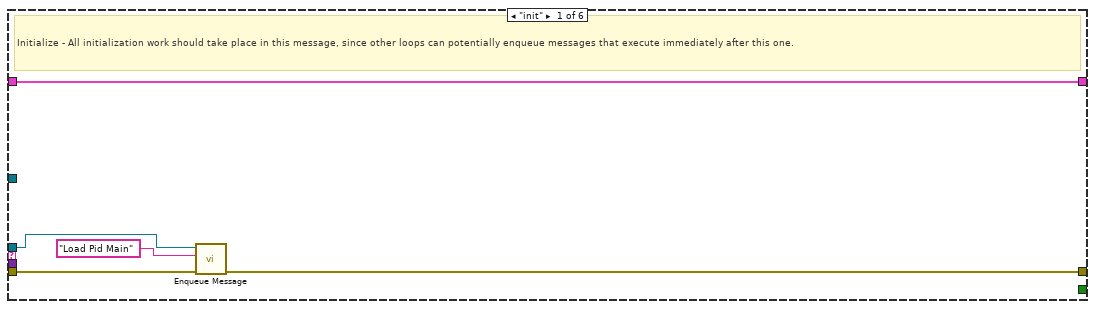
[diagram p8: hidden frame]
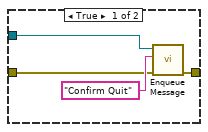
[diagram p9: hidden frame]
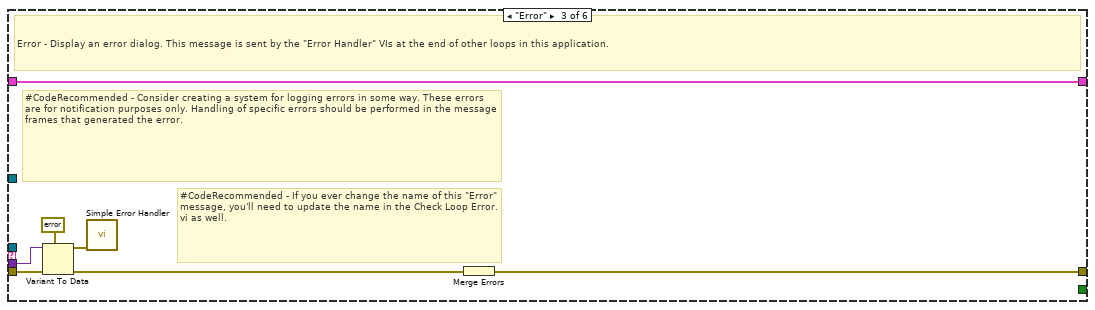
[diagram p10: hidden frame]
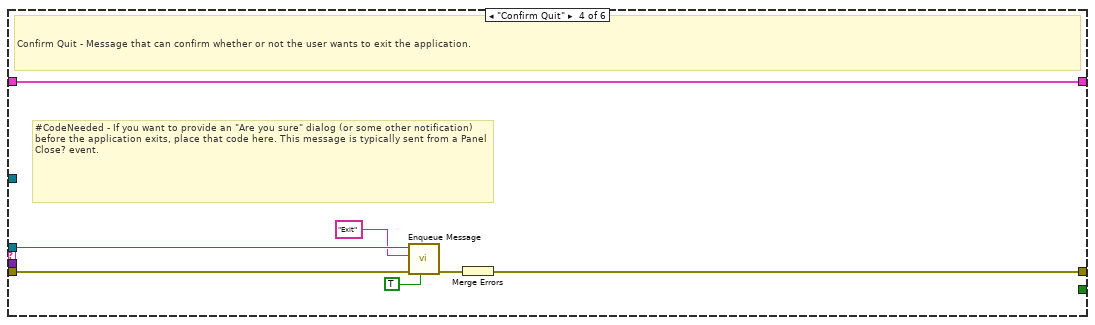
[diagram p11: hidden frame]
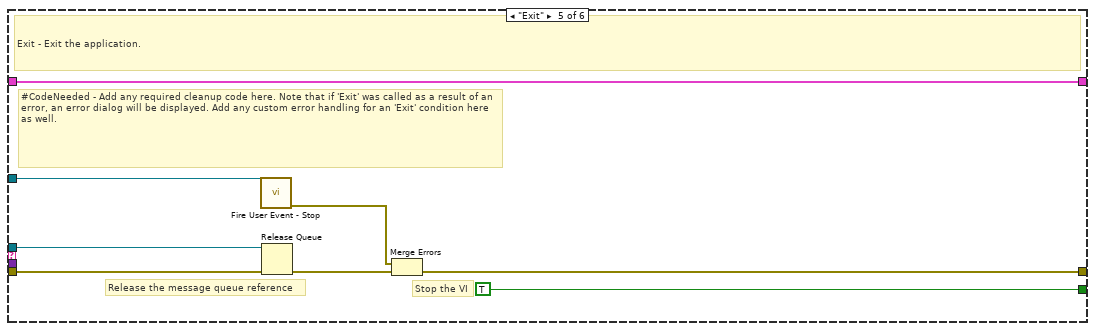
[diagram p12: hidden frame]
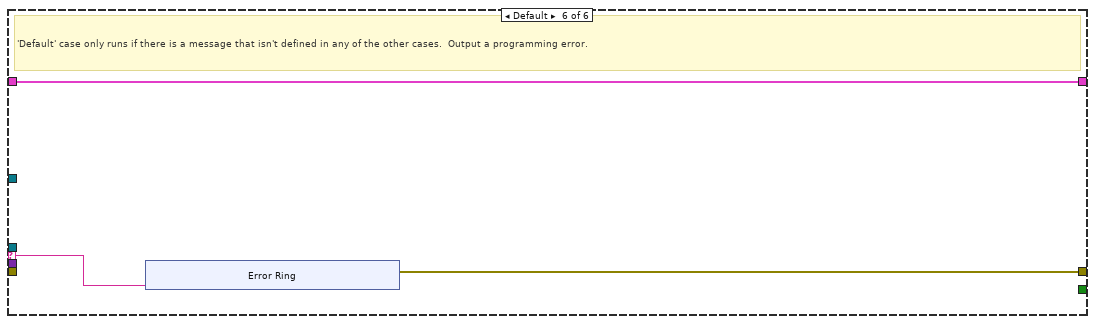
[diagram p13: hidden frame]
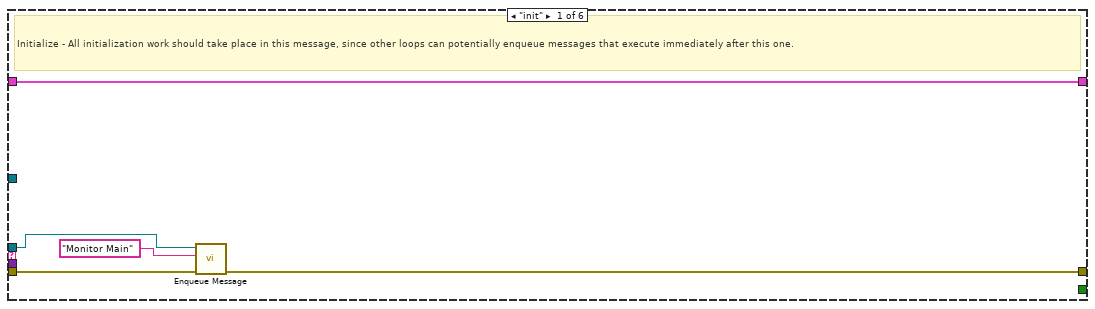
[diagram p14: hidden frame]
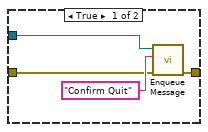
[diagram p15: hidden frame]
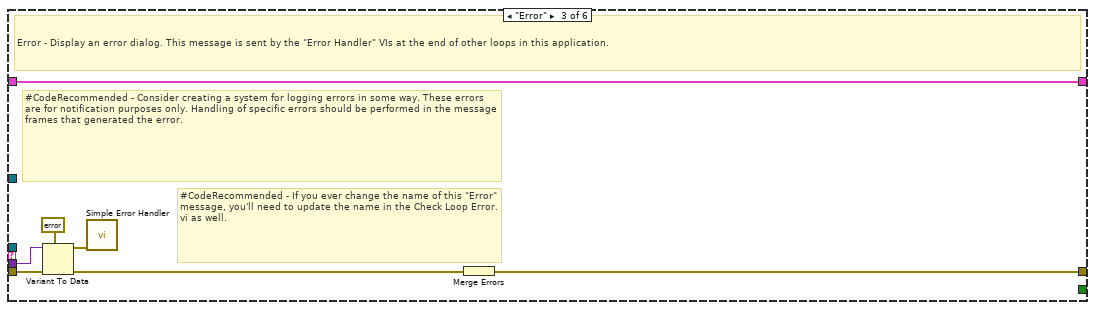
[diagram p16: hidden frame]
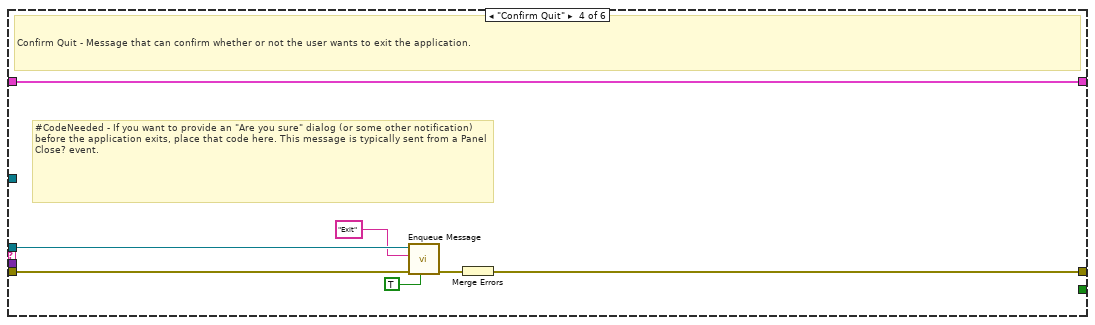
[diagram p17: hidden frame]
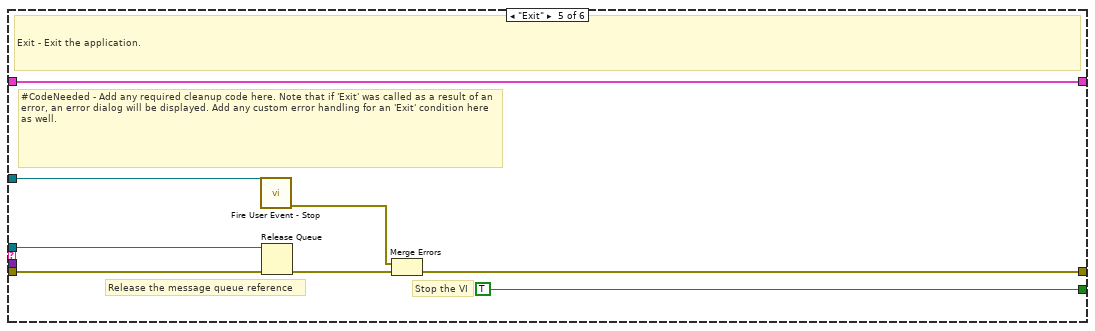
[diagram p18: hidden frame]
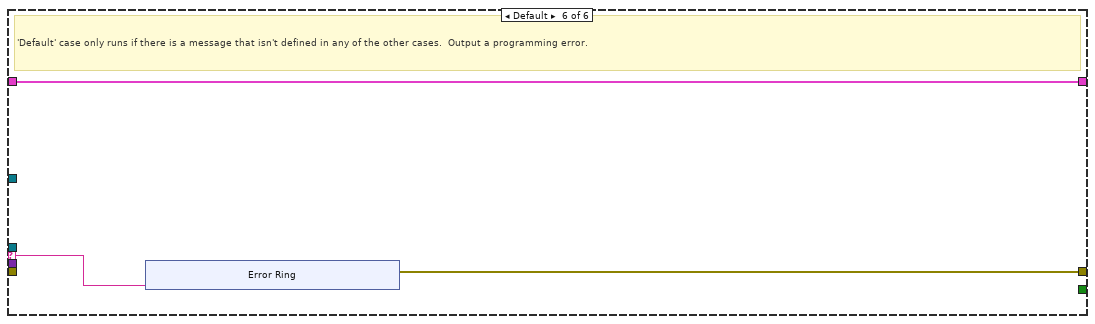
[diagram p19: hidden frame]
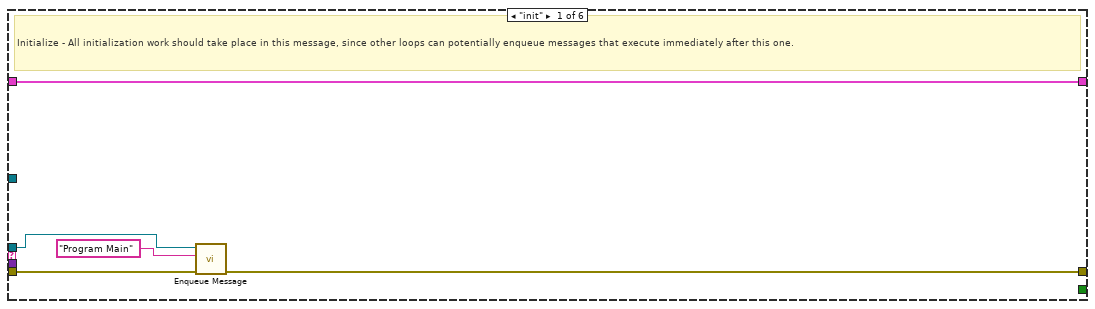
[diagram p20: hidden frame]
diagram:
  n1 = flat-sequence {
    tunnel: [w49] -> w36
    tunnel: T9 {"Main Home Screen"={"GUI"=refnum, "Platform Settings"=refnum, "Configure"=refnum, "Home"=refnum, "EXIT"=refnum, "service 2"=refnum, "MainPage"=refnum, "Analysis"=refnum}, "Platform Settings"={"mm/s  Surge"=refnum, "Update Surge Speed"=refnum, "Drive Error"=refnum, "Disable Axis Jog Soft Limits"=refnum, "mm/s  Sway"=refnum, "Sway and Surge COM Status"=refnum, "Heave COM Status"=refnum, "Enable Platform"=refnum, "Surge Forward Main"=refnum, "Sway Right Main"=refnum, "Sway Left Main"=refnum, "Heave Down Main"=refnum, "Heave Up main"=refnum, "Update Sway Speed"=refnum, "Update Heave Speed"=refnum, "mm/s Heave"=refnum, "mm/sec"=refnum, "mm"=refnum, "Surge Backward Main"=refnum}, "Analysis Screen"={"Analysis Home"=refnum, "Surface Analysis"=refnum, "Imaging"=refnum, "Image Analysis"=refnum, "Post Analysis"=refnum}, "Config Screen"={"Select Load Head"=refnum, "Notes :"=refnum, "FILE"=refnum, "Sample ID :"=refnum, "Operator ID :"=refnum, "Operator Name :"=refnum, "Auto"=refnum}, "Motion Module"={"zNL"=refnum, "NL disp"=refnum, "Rotary Tab"=refnum, "Motion Direction:  3"=refnum, "E.Velocity 2"=refnum, "e.v/ssr 2"=refnum, "Enter Fixed E.Velocity 2"=refnum, "Enter Final SRR 2"=refnum, "Enter initial SRR 2"=refnum, "Enter Fixed SRR 2"=refnum, "Enter the Final E.Velocity (m/s) 2"=refnum, "Enter initial E.Velocity (m/s) 2"=refnum, "Final Speed (RPM) 3"=refnum, "Initial Speed (RPM) 2"=refnum, "Enter the Final Velocity (m/s) 3"=refnum, "Enter initial Velocity (m/s)  3"=refnum, "Ramp Up 2"=refnum, "TEST SELECTION"=refnum, "SPEED SELECTION : "=refnum, "Angular Oscillation Set"=refnum, "Traction"=refnum, "Step Speed"=refnum, "StepTable For Load-Speed"=refnum, "StepTable For Speed"=refnum, "Surge Forward MM"=refnum, "Surge Backward MM"=refnum, "M3 Image"=refnum, "String 39"=refnum, "Sway Left MM"=refnum, "Sway Right MM"=refnum, "Disable Axis Jog Soft Limits"=refnum, "mm"=refnum, "Heave Down MM"=refnum, "Heave Up MM"=refnum, "Wear Track Diameter (mm)"=refnum, "Set WTD"=refnum, "HomeScratch"=refnum, "HomeRot"=refnum, "PlaceModule"=refnum, "Enter the Angle (Deg)"=refnum, "Enter the Frequency (Hz)"=refnum, "Motion Mode:"=refnum, "LR Sway"=refnum, "Rot Hor"=refnum, "Scratch"=refnum, "LR Cam"=refnum, "MMBack"=refnum, "MMNext"=refnum, "Rot Ver"=refnum}, "Environmental control"={"Humidity  Status  3"=refnum, "Low Temp  Status  2"=refnum, "TK4 status 2"=refnum, "Stage Temperature"=refnum, "Sample Temperature"=refnum, "Humidity (Amb)"=refnum, "Clear List"=refnum, "Add to list"=refnum, "Wear"=refnum, "Vibration"=refnum, "Humidity (Chamber)"=refnum, "Temperature (Chamber)"=refnum, "ECR "=refnum, "Temperature (Amb)"=refnum, "Microphone"=refnum, "Acoustic Emission 3"=refnum, "SNext"=refnum, "APBack"=refnum, "Enter the Temperature (°C):"=refnum, "Enter the Stage \nTemperature (°C):"=refnum, "Enter the Humidity (%Rh):"=refnum, "Low Temp"=refnum, "High Temp"=refnum, "Humidity"=refnum, "Sensors Picked"=refnum}, "About Screen"={"Password"=refnum, "Home Service"=refnum, "Advanced Setting"=refnum, "About Tab"=refnum, "ECR Port:"=refnum, "Ramp Port:"=refnum, "Installation/Replacement completed"=refnum, "Loahead"=refnum, "Heave and Surge COM Port:"=refnum, "Sway COM Port:"=refnum, "Temp Modbus:"=refnum, "Humidity Port:"=refnum, "Edit Gain Constants"=refnum, "Save Gain Constants"=refnum}, "Main Screen"={"Main Screen Tab"=refnum, "Angle and Frequency"=refnum, "Stroke (mm)"=refnum, "Angle (Deg)"=refnum, "Main Speed Tab"=refnum, "MTM MOTOR DISPLAY"=refnum, "Disc Speed (m/sec)"=refnum, "Ball Speed (m/sec)"=refnum, "Disc Speed (RPM)"=refnum, "Ball Speed (RPM)"=refnum, "SPEED TAB"=refnum, "Speed (m/sec)"=refnum, "Set Speed (m/sec)"=refnum, "Speed (RPM)"=refnum, "Set Speed"=refnum, "Time Tab"=refnum, "Time ( HH:MM:SS ) 2"=refnum, "Test Duration"=refnum, "Test Duration 4"=refnum, "TEST CYCLE"=refnum, "TOTAL CYCLES"=refnum, "Set Load (N)"=refnum, "Temp Tabs"=refnum, "Heater"=refnum, "TK4 status"=refnum, "ChamberTemp"=refnum, "SetTmp"=refnum, "Controller  Status"=refnum, "ChamberTemp 2"=refnum, "SetTmp 2"=refnum, "Controller  Status 2"=refnum, "ChamberTemp 3"=refnum, "SetTmp 3"=refnum, "Cooling"=refnum, "Load Communication"=refnum, "Ambient \nTemperature"=refnum, "HumCOMStatus"=refnum, "Ambient\n Humidity"=refnum, "Freq (Hz)"=refnum, "Load En"=refnum, "NLt"=refnum, "zNL 2"=refnum, "Humidity On"=refnum, "humidity disp"=refnum, "Set Humidity"=refnum, "NL disp 2"=refnum, "Humidity On 2"=refnum, "humidity disp 2"=refnum, "Set Humidity 2"=refnum, "NL disp 3"=refnum, "AppLoadSeq scratch"=refnum, "Stop Scratch"=refnum, "ClrLog"=refnum, "Trip Log"=refnum, "STOP"=refnum, "Start Test"=refnum, "Test status"=refnum, "AR Led"=refnum, "Data"=refnum, "Health"=refnum, "Sway COM Status"=refnum, "Heave COM Status"=refnum, "Grp Tab"=refnum, "Sub Graph"=refnum, "SD (mm)"=refnum, "Siliding distance Reset Graph"=refnum, "SDGp"=refnum, "Humidity Reset Graph"=refnum, "HumrGp"=refnum, "Acoustic Emission (mV)"=refnum, "Aqucostic Reset Graph"=refnum, "gACQUOS"=refnum, "ECR RESET"=refnum, "ECR"=refnum, "Temperature Reset"=refnum, "Acoustic Emission (mV) 2"=refnum, "Aqucostic Reset Graph 2"=refnum, "gACQUOS 2"=refnum, "ECR RESET 2"=refnum, "ECR 2"=refnum, "Temperature Reset 2"=refnum, "Temperature (deg c)"=refnum, "Speed Reset Graph"=refnum, "Speed Tab"=refnum, "MTM DISC  SPEED"=refnum, "MTM BALL SPEED"=refnum, "speed mm/sec"=refnum, "Hymidity"=refnum, "Humidity Disable trip"=refnum, "CoF Trip  2"=refnum, "Depth Trip"=refnum, "Weart Deapth"=refnum, "Depth Reset Graph"=refnum, "Weart"=refnum, "Depthz"=refnum, "Depth (µm)"=refnum, "WearGp"=refnum, "NL Trip 2"=refnum, "Load pid"=refnum, "Load Disable Trip"=refnum, "Load Reset Graph"=refnum, "NL Display 4"=refnum, "Main Chart 3"=refnum, "BACK"=refnum, "Depth Trip 2"=refnum}, "Loading"={"Indentation"=refnum, "Reference Sample"=refnum, "Load Cell Communication Slide"=refnum, "com 3"=refnum, "com"=refnum, "DecaForce COM Status"=refnum, "Update"=refnum, "Clear 3"=refnum, "seq"=refnum, "Stribeck table"=refnum, "Stribeck Table  For loading"=refnum, "Loading Mode"=refnum, "Enter the Final Load (N)"=refnum, "Enter the CoF Trip"=refnum, "Enter the Friction Force Trip"=refnum, "Enter the Normal load Trip"=refnum, "Enter the Load  (N)"=refnum, "KiloForce"=refnum, "DecaForce "=refnum, "MicroForce"=refnum, "LHBack"=refnum, "LHNext"=refnum, "Enter the Loading Rate (N/min)"=refnum, "Message"=refnum, "Warning 2"=refnum, "SSP 0.75"=refnum, "SSP 0.5"=refnum, "SSP 0.3"=refnum, "Warning"=refnum, "gui GIF"=refnum, "Communication is established"=refnum, "AppLoad 4"=refnum, "Multipoint"=refnum}} ("Data Cluster") -> [w48]
    tunnel: w36 -> [w78]
    tunnel: [w58] -> w35
    tunnel: w35 -> [w85]
    tunnel: [w79] -> w34
    tunnel: w34 -> [w94]
    tunnel: [w93] -> w33
    tunnel: w33 -> [w129]
    tunnel: [w128] -> w31
    tunnel: w31 -> [w180]
    tunnel: [w179] -> w30
    tunnel: w30 -> [w207]
    tunnel: [w206] -> w29
    tunnel: w29 -> [w223]
    tunnel: [w222] -> w28
    tunnel: [w315] -> w6
    tunnel: w28 -> [w316]
    frame #0 {
      n2 = control-ref of="GUI"() -> (w57:refnum<vi>)
      n3 = control-ref of="MainPage"() -> (w51:refnum<vi>)
      n4 = control-ref of="Platform Settings"() -> (w56:refnum<vi>)
      n5 = control-ref of="Configure"() -> (w55:refnum<vi>)
      n6 = control-ref of="Home"() -> (w54:refnum<vi>)
      n7 = control-ref of="EXIT"() -> (w53:refnum<vi>)
      n8 = control-ref of="service 2"() -> (w52:refnum<vi>)
      n9 = control-ref of="Analysis"() -> (w50:refnum<vi>)
      n10 = Bundle By Name(cluster=w48, "Main Home Screen.GUI"=w57, "Main Home Screen.Platform Settings"=w56, "Main Home Screen.Configure"=w55, "Main Home Screen.Home"=w54, "Main Home Screen.EXIT"=w53, "Main Home Screen.service 2"=w52, "Main Home Screen.MainPage"=w51, "Main Home Screen.Analysis"=w50) -> (w49:T9)
    }
    frame #1 {
      n11 = control-ref of="Sway Right Main"() -> (w68:refnum<vi>)
      n12 = control-ref of="Sway Left Main"() -> (w67:refnum<vi>)
      n13 = control-ref of="Heave Down Main"() -> (w66:refnum<vi>)
      n14 = control-ref of="Heave Up main"() -> (w65:refnum<vi>)
      n15 = control-ref of="Update Sway Speed"() -> (w64:refnum<vi>)
      n16 = control-ref of="Update Heave Speed"() -> (w63:refnum<vi>)
      n17 = control-ref of="Surge Backward Main"() -> (w59:refnum<vi>)
      n18 = control-ref of="Update Surge Speed"() -> (w76:refnum<vi>)
      n19 = control-ref of="Disable Axis Jog Soft Limits"() -> (w74:refnum<vi>)
      n20 = control-ref of="Sway and Surge COM Status"() -> (w72:refnum<vi>)
      n21 = control-ref of="Heave COM Status"() -> (w71:refnum<vi>)
      n22 = control-ref of="Enable Platform"() -> (w70:refnum<vi>)
      n23 = control-ref of="Surge Forward Main"() -> (w69:refnum<vi>)
      n24 = control-ref of="mm/s Heave"() -> (w62:refnum<vi>)
      n25 = control-ref of="mm/sec"() -> (w61:refnum<vi>)
      n26 = control-ref of="mm"() -> (w60:refnum<vi>)
      n27 = control-ref of="mm/s  Surge"() -> (w77:refnum<vi>)
      n28 = control-ref of="mm/s  Sway"() -> (w73:refnum<vi>)
      n29 = control-ref of="Drive Error"() -> (w75:refnum<vi>)
      n30 = Bundle By Name(cluster=w78, "Platform Settings.mm/s  Surge"=w77, "Platform Settings.Update Surge Speed"=w76, "Platform Settings.Drive Error"=w75, "Platform Settings.Disable Axis Jog Soft Limits"=w74, "Platform Settings.mm/s  Sway"=w73, "Platform Settings.Sway and Surge COM Status"=w72, "Platform Settings.Heave COM Status"=w71, "Platform Settings.Enable Platform"=w70, "Platform Settings.Surge Forward Main"=w69, "Platform Settings.Sway Right Main"=w68, "Platform Settings.Sway Left Main"=w67, "Platform Settings.Heave Down Main"=w66, "Platform Settings.Heave Up main"=w65, "Platform Settings.Update Sway Speed"=w64, "Platform Settings.Update Heave Speed"=w63, "Platform Settings.mm/s Heave"=w62, "Platform Settings.mm/sec"=w61, "Platform Settings.mm"=w60, "Platform Settings.Surge Backward Main"=w59) -> (w58:T9)
    }
    frame #2 {
      n31 = control-ref of="Analysis Home"() -> (w84:refnum<vi>)
      n32 = control-ref of="Surface Analysis"() -> (w83:refnum<vi>)
      n33 = control-ref of="Imaging"() -> (w82:refnum<vi>)
      n34 = control-ref of="Image Analysis"() -> (w81:refnum<vi>)
      n35 = control-ref of="Post Analysis"() -> (w80:refnum<vi>)
      n36 = Bundle By Name(cluster=w85, "Analysis Screen.Analysis Home"=w84, "Analysis Screen.Surface Analysis"=w83, "Analysis Screen.Imaging"=w82, "Analysis Screen.Image Analysis"=w81, "Analysis Screen.Post Analysis"=w80) -> (w79:T9)
    }
    frame #3 {
      n37 = control-ref of="Select Load Head"() -> (w92:refnum<vi>)
      n38 = control-ref of="Auto"() -> (w86:refnum<vi>)
      n39 = control-ref of="Notes :"() -> (w91:refnum<vi>)
      n40 = control-ref of="FILE"() -> (w90:refnum<vi>)
      n41 = control-ref of="Sample ID :"() -> (w89:refnum<vi>)
      n42 = control-ref of="Operator ID :"() -> (w88:refnum<vi>)
      n43 = control-ref of="Operator Name :"() -> (w87:refnum<vi>)
      n44 = Bundle By Name(cluster=w94, "Config Screen.Select Load Head"=w92, "Config Screen.Notes :"=w91, "Config Screen.FILE"=w90, "Config Screen.Sample ID :"=w89, "Config Screen.Operator ID :"=w88, "Config Screen.Operator Name :"=w87, "Config Screen.Auto"=w86) -> (w93:T9)
    }
    frame #4 {
      n45 = control-ref of="Warning"() -> (w121:refnum<vi>)
      n46 = control-ref of="gui GIF"() -> (w120:refnum<vi>)
      n47 = control-ref of="Warning 2"() -> (w125:refnum<vi>)
      n48 = control-ref of="SSP 0.75"() -> (w124:refnum<vi>)
      n49 = control-ref of="SSP 0.5"() -> (w123:refnum<vi>)
      n50 = control-ref of="SSP 0.3"() -> (w122:refnum<vi>)
      n51 = control-ref of="Communication is established"() -> (w119:refnum<vi>)
      n52 = control-ref of="AppLoad 4"() -> (w118:refnum<vi>)
      n53 = control-ref of="Multipoint"() -> (w117:refnum<vi>)
      n54 = control-ref of="com 3"() -> (w113:refnum<vi>)
      n55 = control-ref of="com"() -> (w112:refnum<vi>)
      n56 = control-ref of="DecaForce COM Status"() -> (w111:refnum<vi>)
      n57 = control-ref of="Update"() -> (w110:refnum<vi>)
      n58 = control-ref of="Clear 3"() -> (w109:refnum<vi>)
      n59 = control-ref of="seq"() -> (w108:refnum<vi>)
      n60 = control-ref of="Stribeck table"() -> (w107:refnum<vi>)
      n61 = control-ref of="KiloForce"() -> (w99:refnum<vi>)
      n62 = control-ref of="DecaForce"() -> (w98:refnum<vi>)
      n63 = control-ref of="MicroForce"() -> (w97:refnum<vi>)
      n64 = control-ref of="LHBack"() -> (w96:refnum<vi>)
      n65 = control-ref of="LHNext"() -> (w95:refnum<vi>)
      n66 = control-ref of="Enter the Loading Rate (N/min)"() -> (w127:refnum<vi>)
      n67 = control-ref of="Enter the Final Load (N)"() -> (w104:refnum<vi>)
      n68 = control-ref of="Enter the CoF Trip"() -> (w103:refnum<vi>)
      n69 = control-ref of="Enter the Friction Force Trip"() -> (w102:refnum<vi>)
      n70 = control-ref of="Enter the Normal load Trip"() -> (w101:refnum<vi>)
      n71 = control-ref of="Enter the Load  (N)"() -> (w100:refnum<vi>)
      n72 = control-ref of="Message"() -> (w126:refnum<vi>)
      n73 = control-ref of="Indentation"() -> (w116:refnum<vi>)
      n74 = control-ref of="Stribeck Table  For loading"() -> (w106:refnum<vi>)
      n75 = control-ref of="Reference Sample"() -> (w115:refnum<vi>)
      n76 = control-ref of="Load Cell Communication Slide"() -> (w114:refnum<vi>)
      n77 = control-ref of="Loading Mode"() -> (w105:refnum<vi>)
      n78 = Bundle By Name(cluster=w129, "Loading.Enter the Loading Rate (N/min)"=w127, "Loading.Message"=w126, "Loading.Warning 2"=w125, "Loading.SSP 0.75"=w124, "Loading.SSP 0.5"=w123, "Loading.SSP 0.3"=w122, "Loading.Warning"=w121, "Loading.gui GIF"=w120, "Loading.Communication is established"=w119, "Loading.AppLoad 4"=w118, "Loading.Multipoint"=w117, "Loading.Indentation"=w116, "Loading.Reference Sample"=w115, "Loading.Load Cell Communication Slide"=w114, "Loading.com 3"=w113, "Loading.com"=w112, "Loading.DecaForce COM Status"=w111, "Loading.Update"=w110, "Loading.Clear 3"=w109, "Loading.seq"=w108, "Loading.Stribeck table"=w107, "Loading.Stribeck Table  For loading"=w106, "Loading.Loading Mode"=w105, "Loading.Enter the Final Load (N)"=w104, "Loading.Enter the CoF Trip"=w103, "Loading.Enter the Friction Force Trip"=w102, "Loading.Enter the Normal load Trip"=w101, "Loading.Enter the Load  (N)"=w100, "Loading.KiloForce"=w99, "Loading.DecaForce"=w98, "Loading.MicroForce"=w97, "Loading.LHBack"=w96, "Loading.LHNext"=w95) -> (w128:T9)
    }
    frame #5 {
      n79 = control-ref of="TEST SELECTION"() -> (w161:refnum<vi>)
      n80 = control-ref of="SPEED SELECTION :"() -> (w160:refnum<vi>)
      n81 = control-ref of="Rotary Tab"() -> (w176:refnum<vi>)
      n82 = control-ref of="e.v/ssr 2"() -> (w173:refnum<vi>)
      n83 = control-ref of="Step Speed"() -> (w157:refnum<vi>)
      n84 = control-ref of="M3 Image"() -> (w152:refnum<vi>)
      n85 = control-ref of="zNL"() -> (w178:refnum<vi>)
      n86 = control-ref of="E.Velocity 2"() -> (w174:refnum<vi>)
      n87 = control-ref of="Ramp Up 2"() -> (w162:refnum<vi>)
      n88 = control-ref of="Angular Oscillation Set"() -> (w159:refnum<vi>)
      n89 = control-ref of="Traction"() -> (w158:refnum<vi>)
      n90 = control-ref of="Surge Forward MM"() -> (w154:refnum<vi>)
      n91 = control-ref of="Surge Backward MM"() -> (w153:refnum<vi>)
      n92 = control-ref of="Sway Left MM"() -> (w150:refnum<vi>)
      n93 = control-ref of="Sway Right MM"() -> (w149:refnum<vi>)
      n94 = control-ref of="Disable Axis Jog Soft Limits"() -> (w148:refnum<vi>)
      n95 = control-ref of="Heave Down MM"() -> (w146:refnum<vi>)
      n96 = control-ref of="Heave Up MM"() -> (w145:refnum<vi>)
      n97 = control-ref of="Set WTD"() -> (w143:refnum<vi>)
      n98 = control-ref of="HomeScratch"() -> (w142:refnum<vi>)
      n99 = control-ref of="HomeRot"() -> (w141:refnum<vi>)
      n100 = control-ref of="PlaceModule"() -> (w140:refnum<vi>)
      n101 = control-ref of="LR Sway"() -> (w136:refnum<vi>)
      n102 = control-ref of="Rot Hor"() -> (w135:refnum<vi>)
      n103 = control-ref of="Scratch"() -> (w134:refnum<vi>)
      n104 = control-ref of="LR Cam"() -> (w133:refnum<vi>)
      n105 = control-ref of="MMBack"() -> (w132:refnum<vi>)
      n106 = control-ref of="MMNext"() -> (w131:refnum<vi>)
      n107 = control-ref of="Rot Ver"() -> (w130:refnum<vi>)
      n108 = control-ref of="NL disp"() -> (w177:refnum<vi>)
      n109 = control-ref of="Enter Fixed E.Velocity 2"() -> (w172:refnum<vi>)
      n110 = control-ref of="Enter Final SRR 2"() -> (w171:refnum<vi>)
      n111 = control-ref of="Enter initial SRR 2"() -> (w170:refnum<vi>)
      n112 = control-ref of="Enter Fixed SRR 2"() -> (w169:refnum<vi>)
      n113 = control-ref of="Enter the Final E.Velocity (m/s) 2"() -> (w168:refnum<vi>)
      n114 = control-ref of="Enter initial E.Velocity (m/s) 2"() -> (w167:refnum<vi>)
      n115 = control-ref of="Final Speed (RPM) 3"() -> (w166:refnum<vi>)
      n116 = control-ref of="Initial Speed (RPM) 2"() -> (w165:refnum<vi>)
      n117 = control-ref of="Enter the Final Velocity (m/s) 3"() -> (w164:refnum<vi>)
      n118 = control-ref of="Enter initial Velocity (m/s)  3"() -> (w163:refnum<vi>)
      n119 = control-ref of="mm"() -> (w147:refnum<vi>)
      n120 = control-ref of="Wear Track Diameter (mm)"() -> (w144:refnum<vi>)
      n121 = control-ref of="Enter the Angle (Deg)"() -> (w139:refnum<vi>)
      n122 = control-ref of="Enter the Frequency (Hz)"() -> (w138:refnum<vi>)
      n123 = control-ref of="String 39"() -> (w151:refnum<vi>)
      n124 = control-ref of="StepTable For Load-Speed"() -> (w156:refnum<vi>)
      n125 = control-ref of="StepTable For Speed"() -> (w155:refnum<vi>)
      n126 = control-ref of="Motion Direction:  3"() -> (w175:refnum<vi>)
      n127 = control-ref of="Motion Mode:"() -> (w137:refnum<vi>)
      n128 = Bundle By Name(cluster=w180, "Motion Module.zNL"=w178, "Motion Module.NL disp"=w177, "Motion Module.Rotary Tab"=w176, "Motion Module.Motion Direction:  3"=w175, "Motion Module.E.Velocity 2"=w174, "Motion Module.e.v/ssr 2"=w173, "Motion Module.Enter Fixed E.Velocity 2"=w172, "Motion Module.Enter Final SRR 2"=w171, "Motion Module.Enter initial SRR 2"=w170, "Motion Module.Enter Fixed SRR 2"=w169, "Motion Module.Enter the Final E.Velocity (m/s) 2"=w168, "Motion Module.Enter initial E.Velocity (m/s) 2"=w167, "Motion Module.Final Speed (RPM) 3"=w166, "Motion Module.Initial Speed (RPM) 2"=w165, "Motion Module.Enter the Final Velocity (m/s) 3"=w164, "Motion Module.Enter initial Velocity (m/s)  3"=w163, "Motion Module.Ramp Up 2"=w162, "Motion Module.TEST SELECTION"=w161, "Motion Module.SPEED SELECTION :"=w160, "Motion Module.Angular Oscillation Set"=w159, "Motion Module.Traction"=w158, "Motion Module.Step Speed"=w157, "Motion Module.StepTable For Load-Speed"=w156, "Motion Module.StepTable For Speed"=w155, "Motion Module.Surge Forward MM"=w154, "Motion Module.Surge Backward MM"=w153, "Motion Module.M3 Image"=w152, "Motion Module.String 39"=w151, "Motion Module.Sway Left MM"=w150, "Motion Module.Sway Right MM"=w149, "Motion Module.Disable Axis Jog Soft Limits"=w148, "Motion Module.mm"=w147, "Motion Module.Heave Down MM"=w146, "Motion Module.Heave Up MM"=w145, "Motion Module.Wear Track Diameter (mm)"=w144, "Motion Module.Set WTD"=w143, "Motion Module.HomeScratch"=w142, "Motion Module.HomeRot"=w141, "Motion Module.PlaceModule"=w140, "Motion Module.Enter the Angle (Deg)"=w139, "Motion Module.Enter the Frequency (Hz)"=w138, "Motion Module.Motion Mode:"=w137, "Motion Module.LR Sway"=w136, "Motion Module.Rot Hor"=w135, "Motion Module.Scratch"=w134, "Motion Module.LR Cam"=w133, "Motion Module.MMBack"=w132, "Motion Module.MMNext"=w131, "Motion Module.Rot Ver"=w130) -> (w179:T9)
    }
    frame #6 {
      n129 = control-ref of="Add to list"() -> (w198:refnum<vi>)
      n130 = control-ref of="Wear"() -> (w197:refnum<vi>)
      n131 = control-ref of="Vibration"() -> (w196:refnum<vi>)
      n132 = control-ref of="Humidity (Chamber)"() -> (w195:refnum<vi>)
      n133 = control-ref of="Temperature (Chamber)"() -> (w194:refnum<vi>)
      n134 = control-ref of="ECR"() -> (w193:refnum<vi>)
      n135 = control-ref of="Temperature (Amb)"() -> (w192:refnum<vi>)
      n136 = control-ref of="Microphone"() -> (w191:refnum<vi>)
      n137 = control-ref of="Acoustic Emission 3"() -> (w190:refnum<vi>)
      n138 = control-ref of="SNext"() -> (w189:refnum<vi>)
      n139 = control-ref of="APBack"() -> (w188:refnum<vi>)
      n140 = control-ref of="Low Temp"() -> (w184:refnum<vi>)
      n141 = control-ref of="High Temp"() -> (w183:refnum<vi>)
      n142 = control-ref of="Humidity"() -> (w182:refnum<vi>)
      n143 = control-ref of="Humidity  Status  3"() -> (w205:refnum<vi>)
      n144 = control-ref of="Low Temp  Status  2"() -> (w204:refnum<vi>)
      n145 = control-ref of="TK4 status 2"() -> (w203:refnum<vi>)
      n146 = control-ref of="Humidity (Amb)"() -> (w200:refnum<vi>)
      n147 = control-ref of="Clear List"() -> (w199:refnum<vi>)
      n148 = control-ref of="Enter the Temperature (°C):"() -> (w187:refnum<vi>)
      n149 = control-ref of="Enter the Stage \nTemperature (°C):"() -> (w186:refnum<vi>)
      n150 = control-ref of="Enter the Humidity (%Rh):"() -> (w185:refnum<vi>)
      n151 = control-ref of="Sensors Picked"() -> (w181:refnum<vi>)
      n152 = control-ref of="Stage Temperature"() -> (w202:refnum<vi>)
      n153 = control-ref of="Sample Temperature"() -> (w201:refnum<vi>)
      n154 = Bundle By Name(cluster=w207, "Environmental control.Humidity  Status  3"=w205, "Environmental control.Low Temp  Status  2"=w204, "Environmental control.TK4 status 2"=w203, "Environmental control.Stage Temperature"=w202, "Environmental control.Sample Temperature"=w201, "Environmental control.Humidity (Amb)"=w200, "Environmental control.Clear List"=w199, "Environmental control.Add to list"=w198, "Environmental control.Wear"=w197, "Environmental control.Vibration"=w196, "Environmental control.Humidity (Chamber)"=w195, "Environmental control.Temperature (Chamber)"=w194, "Environmental control.ECR"=w193, "Environmental control.Temperature (Amb)"=w192, "Environmental control.Microphone"=w191, "Environmental control.Acoustic Emission 3"=w190, "Environmental control.SNext"=w189, "Environmental control.APBack"=w188, "Environmental control.Enter the Temperature (°C):"=w187, "Environmental control.Enter the Stage \nTemperature (°C):"=w186, "Environmental control.Enter the Humidity (%Rh):"=w185, "Environmental control.Low Temp"=w184, "Environmental control.High Temp"=w183, "Environmental control.Humidity"=w182, "Environmental control.Sensors Picked"=w181) -> (w206:T9)
    }
    frame #7 {
      n155 = control-ref of="ECR Port:"() -> (w217:refnum<vi>)
      n156 = control-ref of="Ramp Port:"() -> (w216:refnum<vi>)
      n157 = control-ref of="Heave and Surge COM Port:"() -> (w213:refnum<vi>)
      n158 = control-ref of="Sway COM Port:"() -> (w212:refnum<vi>)
      n159 = control-ref of="Temp Modbus:"() -> (w211:refnum<vi>)
      n160 = control-ref of="Humidity Port:"() -> (w210:refnum<vi>)
      n161 = control-ref of="About Tab"() -> (w218:refnum<vi>)
      n162 = control-ref of="Home Service"() -> (w220:refnum<vi>)
      n163 = control-ref of="Advanced Setting"() -> (w219:refnum<vi>)
      n164 = control-ref of="Installation/Replacement completed"() -> (w215:refnum<vi>)
      n165 = control-ref of="Loahead"() -> (w214:refnum<vi>)
      n166 = control-ref of="Edit Gain Constants"() -> (w209:refnum<vi>)
      n167 = control-ref of="Save Gain Constants"() -> (w208:refnum<vi>)
      n168 = control-ref of="Password"() -> (w221:refnum<vi>)
      n169 = Bundle By Name(cluster=w223, "About Screen.Password"=w221, "About Screen.Home Service"=w220, "About Screen.Advanced Setting"=w219, "About Screen.About Tab"=w218, "About Screen.ECR Port:"=w217, "About Screen.Ramp Port:"=w216, "About Screen.Installation/Replacement completed"=w215, "About Screen.Loahead"=w214, "About Screen.Heave and Surge COM Port:"=w213, "About Screen.Sway COM Port:"=w212, "About Screen.Temp Modbus:"=w211, "About Screen.Humidity Port:"=w210, "About Screen.Edit Gain Constants"=w209, "About Screen.Save Gain Constants"=w208) -> (w222:T9)
    }
    frame #8 {
      n170 = control-ref of="SDGp"() -> (w255:refnum<vi>)
      n171 = control-ref of="HumrGp"() -> (w253:refnum<vi>)
      n172 = control-ref of="gACQUOS"() -> (w250:refnum<vi>)
      n173 = control-ref of="ECR"() -> (w248:refnum<vi>)
      n174 = control-ref of="Temperature (deg c)"() -> (w246:refnum<vi>)
      n175 = control-ref of="MTM DISC  SPEED"() -> (w243:refnum<vi>)
      n176 = control-ref of="MTM BALL SPEED"() -> (w242:refnum<vi>)
      n177 = control-ref of="speed mm/sec"() -> (w241:refnum<vi>)
      n178 = control-ref of="WearGp"() -> (w231:refnum<vi>)
      n179 = control-ref of="Main Chart 3"() -> (w225:refnum<vi>)
      n180 = control-ref of="Main Screen Tab"() -> (w314:refnum<vi>)
      n181 = control-ref of="Angle and Frequency"() -> (w313:refnum<vi>)
      n182 = control-ref of="Main Speed Tab"() -> (w310:refnum<vi>)
      n183 = control-ref of="MTM MOTOR DISPLAY"() -> (w309:refnum<vi>)
      n184 = control-ref of="SPEED TAB"() -> (w304:refnum<vi>)
      n185 = control-ref of="Time Tab"() -> (w299:refnum<vi>)
      n186 = control-ref of="Temp Tabs"() -> (w292:refnum<vi>)
      n187 = control-ref of="Grp Tab"() -> (w259:refnum<vi>)
      n188 = control-ref of="Sub Graph"() -> (w258:refnum<vi>)
      n189 = control-ref of="Speed Tab"() -> (w244:refnum<vi>)
      n190 = control-ref of="Heater"() -> (w291:refnum<vi>)
      n191 = control-ref of="TK4 status"() -> (w290:refnum<vi>)
      n192 = control-ref of="Controller  Status"() -> (w287:refnum<vi>)
      n193 = control-ref of="Cooling"() -> (w284:refnum<vi>)
      n194 = control-ref of="Load Communication"() -> (w283:refnum<vi>)
      n195 = control-ref of="HumCOMStatus"() -> (w281:refnum<vi>)
      n196 = control-ref of="Load En"() -> (w278:refnum<vi>)
      n197 = control-ref of="NLt"() -> (w277:refnum<vi>)
      n198 = control-ref of="zNL 2"() -> (w276:refnum<vi>)
      n199 = control-ref of="Humidity On"() -> (w275:refnum<vi>)
      n200 = control-ref of="AppLoadSeq scratch"() -> (w271:refnum<vi>)
      n201 = control-ref of="Stop Scratch"() -> (w270:refnum<vi>)
      n202 = control-ref of="ClrLog"() -> (w269:refnum<vi>)
      n203 = control-ref of="STOP"() -> (w267:refnum<vi>)
      n204 = control-ref of="Start Test"() -> (w266:refnum<vi>)
      n205 = control-ref of="Test status"() -> (w265:refnum<vi>)
      n206 = control-ref of="AR Led"() -> (w264:refnum<vi>)
      n207 = control-ref of="Data"() -> (w263:refnum<vi>)
      n208 = control-ref of="Health"() -> (w262:refnum<vi>)
      n209 = control-ref of="Sway COM Status"() -> (w261:refnum<vi>)
      n210 = control-ref of="Heave COM Status"() -> (w260:refnum<vi>)
      n211 = control-ref of="Siliding distance Reset Graph"() -> (w256:refnum<vi>)
      n212 = control-ref of="Humidity Reset Graph"() -> (w254:refnum<vi>)
      n213 = control-ref of="Aqucostic Reset Graph"() -> (w251:refnum<vi>)
      n214 = control-ref of="ECR RESET"() -> (w249:refnum<vi>)
      n215 = control-ref of="Temperature Reset"() -> (w247:refnum<vi>)
      n216 = control-ref of="Speed Reset Graph"() -> (w245:refnum<vi>)
      n217 = control-ref of="Hymidity"() -> (w240:refnum<vi>)
      n218 = control-ref of="Humidity Disable trip"() -> (w239:refnum<vi>)
      n219 = control-ref of="Weart Deapth"() -> (w236:refnum<vi>)
      n220 = control-ref of="Depth Reset Graph"() -> (w235:refnum<vi>)
      n221 = control-ref of="Weart"() -> (w234:refnum<vi>)
      n222 = control-ref of="Depthz"() -> (w233:refnum<vi>)
      n223 = control-ref of="Load pid"() -> (w229:refnum<vi>)
      n224 = control-ref of="Load Disable Trip"() -> (w228:refnum<vi>)
      n225 = control-ref of="Load Reset Graph"() -> (w227:refnum<vi>)
      n226 = control-ref of="BACK"() -> (w224:refnum<vi>)
      n227 = control-ref of="Depth Trip"() -> ()  [unwired: 1 out]
      n228 = control-ref of="Stroke (mm)"() -> (w312:refnum<vi>)
      n229 = control-ref of="Angle (Deg)"() -> (w311:refnum<vi>)
      n230 = control-ref of="Disc Speed (m/sec)"() -> (w308:refnum<vi>)
      n231 = control-ref of="Ball Speed (m/sec)"() -> (w307:refnum<vi>)
      n232 = control-ref of="Disc Speed (RPM)"() -> (w306:refnum<vi>)
      n233 = control-ref of="Ball Speed (RPM)"() -> (w305:refnum<vi>)
      n234 = control-ref of="Speed (m/sec)"() -> (w303:refnum<vi>)
      n235 = control-ref of="Set Speed (m/sec)"() -> (w302:refnum<vi>)
      n236 = control-ref of="Speed (RPM)"() -> (w301:refnum<vi>)
      n237 = control-ref of="Set Speed"() -> (w300:refnum<vi>)
      n238 = control-ref of="Time ( HH:MM:SS ) 2"() -> (w298:refnum<vi>)
      n239 = control-ref of="Test Duration"() -> (w297:refnum<vi>)
      n240 = control-ref of="Test Duration 4"() -> (w296:refnum<vi>)
      n241 = control-ref of="TEST CYCLE"() -> (w295:refnum<vi>)
      n242 = control-ref of="TOTAL CYCLES"() -> (w294:refnum<vi>)
      n243 = control-ref of="Set Load (N)"() -> (w293:refnum<vi>)
      n244 = control-ref of="ChamberTemp"() -> (w289:refnum<vi>)
      n245 = control-ref of="SetTmp"() -> (w288:refnum<vi>)
      n246 = control-ref of="ChamberTemp"() -> (w286:refnum<vi>)
      n247 = control-ref of="SetTmp"() -> (w285:refnum<vi>)
      n248 = control-ref of="Ambient \nTemperature"() -> (w282:refnum<vi>)
      n249 = control-ref of="Ambient\n Humidity"() -> (w280:refnum<vi>)
      n250 = control-ref of="Freq (Hz)"() -> (w279:refnum<vi>)
      n251 = control-ref of="humidity disp"() -> (w274:refnum<vi>)
      n252 = control-ref of="Set Humidity"() -> (w273:refnum<vi>)
      n253 = control-ref of="NL disp 2"() -> (w272:refnum<vi>)
      n254 = control-ref of="SD (mm)"() -> (w257:refnum<vi>)
      n255 = control-ref of="Acoustic Emission (mV)"() -> (w252:refnum<vi>)
      n256 = control-ref of="CoF Trip  2"() -> (w238:refnum<vi>)
      n257 = control-ref of="Depth Trip"() -> (w237:refnum<vi>)
      n258 = control-ref of="Depth (µm)"() -> (w232:refnum<vi>)
      n259 = control-ref of="NL Trip 2"() -> (w230:refnum<vi>)
      n260 = control-ref of="NL Display 4"() -> (w226:refnum<vi>)
      n261 = control-ref of="Trip Log"() -> (w268:refnum<vi>)
      n262 = Bundle By Name(cluster=w316, "Main Screen.Main Screen Tab"=w314, "Main Screen.Angle and Frequency"=w313, "Main Screen.Stroke (mm)"=w312, "Main Screen.Angle (Deg)"=w311, "Main Screen.Main Speed Tab"=w310, "Main Screen.MTM MOTOR DISPLAY"=w309, "Main Screen.Disc Speed (m/sec)"=w308, "Main Screen.Ball Speed (m/sec)"=w307, "Main Screen.Disc Speed (RPM)"=w306, "Main Screen.Ball Speed (RPM)"=w305, "Main Screen.SPEED TAB"=w304, "Main Screen.Speed (m/sec)"=w303, "Main Screen.Set Speed (m/sec)"=w302, "Main Screen.Speed (RPM)"=w301, "Main Screen.Set Speed"=w300, "Main Screen.Time Tab"=w299, "Main Screen.Time ( HH:MM:SS ) 2"=w298, "Main Screen.Test Duration"=w297, "Main Screen.Test Duration 4"=w296, "Main Screen.TEST CYCLE"=w295, "Main Screen.TOTAL CYCLES"=w294, "Main Screen.Set Load (N)"=w293, "Main Screen.Temp Tabs"=w292, "Main Screen.Heater"=w291, "Main Screen.TK4 status"=w290, "Main Screen.ChamberTemp"=w289, "Main Screen.SetTmp"=w288, "Main Screen.Controller  Status"=w287, "Main Screen.ChamberTemp 2"=w286, "Main Screen.SetTmp 2"=w285, "Main Screen.Cooling"=w284, "Main Screen.Load Communication"=w283, "Main Screen.Ambient \nTemperature"=w282, "Main Screen.HumCOMStatus"=w281, "Main Screen.Ambient\n Humidity"=w280, "Main Screen.Freq (Hz)"=w279, "Main Screen.Load En"=w278, "Main Screen.NLt"=w277, "Main Screen.zNL 2"=w276, "Main Screen.Humidity On"=w275, "Main Screen.humidity disp"=w274, "Main Screen.Set Humidity"=w273, "Main Screen.NL disp 2"=w272, "Main Screen.AppLoadSeq scratch"=w271, "Main Screen.Stop Scratch"=w270, "Main Screen.ClrLog"=w269, "Main Screen.Trip Log"=w268, "Main Screen.STOP"=w267, "Main Screen.Start Test"=w266, "Main Screen.Test status"=w265, "Main Screen.AR Led"=w264, "Main Screen.Data"=w263, "Main Screen.Health"=w262, "Main Screen.Sway COM Status"=w261, "Main Screen.Heave COM Status"=w260, "Main Screen.Grp Tab"=w259, "Main Screen.Sub Graph"=w258, "Main Screen.SD (mm)"=w257, "Main Screen.Siliding distance Reset Graph"=w256, "Main Screen.SDGp"=w255, "Main Screen.Humidity Reset Graph"=w254, "Main Screen.HumrGp"=w253, "Main Screen.Acoustic Emission (mV)"=w252, "Main Screen.Aqucostic Reset Graph"=w251, "Main Screen.gACQUOS"=w250, "Main Screen.ECR RESET"=w249, "Main Screen.ECR"=w248, "Main Screen.Temperature Reset"=w247, "Main Screen.Temperature (deg c)"=w246, "Main Screen.Speed Reset Graph"=w245, "Main Screen.Speed Tab"=w244, "Main Screen.MTM DISC  SPEED"=w243, "Main Screen.MTM BALL SPEED"=w242, "Main Screen.speed mm/sec"=w241, "Main Screen.Hymidity"=w240, "Main Screen.Humidity Disable trip"=w239, "Main Screen.CoF Trip  2"=w238, "Main Screen.Depth Trip"=w237, "Main Screen.Weart Deapth"=w236, "Main Screen.Depth Reset Graph"=w235, "Main Screen.Weart"=w234, "Main Screen.Depthz"=w233, "Main Screen.Depth (µm)"=w232, "Main Screen.WearGp"=w231, "Main Screen.NL Trip 2"=w230, "Main Screen.Load pid"=w229, "Main Screen.Load Disable Trip"=w228, "Main Screen.Load Reset Graph"=w227, "Main Screen.NL Display 4"=w226, "Main Screen.Main Chart 3"=w225, "Main Screen.BACK"=w224) -> (w315:T9)
    }
  }
  n263 = call <userlib>:"Fit VI window to Largest Dec.vi"() -> ("error out"=w24:errorcluster, "dup VI Ref"=w21:refnum<vi>)  [unwired: 6 in]
  n264 = invoke on="Invoke Node" class="VI" method="FP.Run-Time Position.Maximized"(reference=w21, error in=w24) -> (error out=w23:errorcluster)  [unwired: 2 in, 3 out]
  n265 = call <vilib>:"Clear Errors.vi"("error in (no error)"=w23) -> ("error out"=w22:errorcluster)  [unwired: 5 in, 1 out]
  n266 = control-ref of="This VI"() -> (w27:refnum<vi>)
  n267 = invoke on="Invoke Node" class="VI" method="Default Vals.Reinit All"(reference=w27, error in=w22) -> (reference out=w25:refnum<vi>, error out=w26:errorcluster)  [unwired: 1 in, 1 out]
  n268 = Close Reference(reference=w25, error in (no error)=w26) -> (error out=w20:errorcluster)
  n269 = call "Create User Event - Stop.vi"("error in (no error)"=w20) -> ("error out"=w4:errorcluster, "User Event - Stop"=w5:refnum<user-event>)  [unwired: 9 in]
  n270 = call "main screen queue out Unitest.vi"("error in (no error)"=w4) -> ("error out"=w47:errorcluster, "output Queue"=w19:T10)  [unwired: 9 in]
  n271 = Unbundle By Name(w19) -> ("UI Loop"=w45:refnum<queue>)
  n272 = Unbundle By Name(w19) -> ("LOAD COM LOOP"=w17:refnum<queue>)
  n273 = Unbundle By Name(w19) -> ("SWAY MOTOR COM LOOP"=w16:refnum<queue>)
  n274 = Unbundle By Name(w19) -> ("HEAVE MOTOR COM LOOP"=w14:refnum<queue>)
  n275 = Unbundle By Name(w19) -> ("TEMPERATURE COM LOOP"=w13:refnum<queue>)
  n276 = Unbundle By Name(w19) -> ("RAMP MOTOR COM LOOP"=w10:refnum<queue>)
  n277 = Unbundle By Name(w19) -> ("ECR PORT"=w9:refnum<queue>)
  n278 = Unbundle By Name(w19) -> ("HUMIDITY COM PORT"=w8:refnum<queue>)
  n279 = Unbundle By Name(w19) -> ("PROGRAM LOOP"=w7:refnum<queue>)
  n280 = Unbundle By Name(w19) -> ("MONITOR LOOP"=w3:refnum<queue>)
  n281 = Unbundle By Name(w19) -> ("LOAD PID"=w2:refnum<queue>)
  n282 = Unbundle By Name(w19) -> ("REPORT"=w1:refnum<queue>)
  n283 = register-events(w5) -> (reference out=w39:refnum<event-registration>, error out=w37:errorcluster)  [unwired: 2 in]
  n284 = Merge Errors(w37, w47) -> (w38:errorcluster)
  n285 = while {
    tunnel: w45 -> [w324]
    shift-right: [w322] -> w42
    shift-left: w39 -> [w323]
    tunnel: [w318] -> w40
    stop <- w320 stop-if-true
    # "Event Handling Loop"
    n286 = event shown="[4] <User Event - Stop>: User Event" {
      selector: w323 -> [_ _ _ _ _]
      dyn-events: [_ _ _ _ _] -> w322
      timeout: 100 -> [_ _ _ _ _]
      tunnel: [_ _ _ _ TRUE ("Discard?")] -> w320
      tunnel: w324 -> [w329 w333 w336 w341 w343]
      tunnel: [w328 w331 _ w340 _] -> w321
      tunnel: [w327 w332 w336 w339 w343] -> w319
      event Panel Close? {
        n287 = event-data() -> ()  [unwired: 1 in, 1 out]
        n288 = call-poly "Enqueue Message.vi"("Priority Message? (F)"=TRUE, "Message"="Confirm Quit", "Message Queue"=w329) -> ("error out"=w328:errorcluster, "dup Message Queue"=w327:refnum<queue>)  [unwired: 7 in]
        n289 = event-data("Discard?"=TRUE) -> ()  [unwired: 1 in, 1 out]
      }
      event Timeout {
        n290 = event-data() -> ()  [unwired: 1 in, 1 out]
        n291 = call-poly "Enqueue Message.vi"("Priority Message? (F)"=TRUE, "Message"="Time Out", "Message Queue"=w333) -> ("error out"=w331:errorcluster, "dup Message Queue"=w332:refnum<queue>)  [unwired: 7 in]
      }
      event Application Instance Close {
        # "#CodeRecommended - When a project closes, all VIs within that project are aborted and leave memory. However, any code placed in this event frame is guaranteed to run to completion, so add any cleanup code that absolutely must happen here."
        n292 = event-data() -> ()  [unwired: 1 in, 1 out]
      }
      event "EXIT": Value Change {
        n293 = event-data() -> ()  [unwired: 1 in, 1 out]
        n294 = call-poly "Enqueue Message.vi"("Priority Message? (F)"=TRUE, "Message"="Exit", "Message Queue"=w341) -> ("error out"=w340:errorcluster, "dup Message Queue"=w339:refnum<queue>)  [unwired: 7 in]
      }
      event User Event {
        # "The Message Handling Loop processed an \"Exit\" message, which fired this event to stop the Event Handling Loop."
        n295 = event-data() -> ()  [unwired: 1 in, 1 out]
      }
    }
    n296 = call "LAB-IQ Error Handler - Event Handling Loop.vi"("error in (no error)"=w321, "Message Queue"=w319) -> ("dup error in"=w318:errorcluster)  [unwired: 8 in, 1 out]
  }
  n297 = while {
    shift-right: [w354] -> _
    shift-left: w6 -> [w355]
    tunnel: [w348] -> w18
    tunnel: w17 -> [w346]
    tunnel: w4 -> [w345]
    tunnel: w5 -> [w344]
    stop <- w353 stop-if-true
    # "Load  Handling Loop"
    n298 = call "Dequeue Message.vi"("error in (no error)"=w345, "Message Queue"=w346) -> ("error out"=w352:errorcluster, "Message Data"=w350:variant, "Message"=w351:string, "dup Message Queue"=w349:refnum<queue>)  [unwired: 6 in]
    n299 = case "Message Cases" shown="\"Exit\"" w351 {
      selector: w351 -> [_ _ _ _ _ w399]
      tunnel: w349 -> [w356 w367 _ w386 w398 _]
      tunnel: w352 -> [w359 w364 w383 w390 w392 _]
      tunnel: [w360 w368 w377 w388 w394 w400] -> w347
      tunnel: w355 -> [w358 w366 w382 w389 w397 w401]
      tunnel: [w358 w366 w382 w389 w397 w401] -> w354
      tunnel: [_ _ _ _ TRUE _] -> w353
      tunnel: w350 -> [_ _ w381 _ _ _]
      tunnel: w344 -> [_ _ _ _ w391 _]
      frame "init" {
        # "Bundle control references and a sample string value."
        # "Initialize - All initialization work should take place in this message, since other loops can potentially enqueue messages that execute immediately after this one."
        n300 = call-poly "Enqueue Message.vi"("error in (no error)"=w359, "Message"="Load Main", "Message Queue"=w356) -> ("error out"=w360:errorcluster)  [unwired: 7 in, 1 out]
      }
      frame "Load Main" {
        n301 = Unbundle By Name(w366) -> ("Main Home Screen.EXIT"=w365:refnum<vi>)
        n302 = property class="Bool (strict)"(reference=w365) -> (reference out=w362:refnum<vi>, error out=w363:errorcluster, "Value"=w361:bool)  [unwired: 1 in]
        n303 = Close Reference(reference=w362, error in (no error)=w363) -> ()  [unwired: 1 out]
        n304 = case shown="False" w361 {
          tunnel: [w371 w375] -> w368
          tunnel: w367 -> [w370 w374]
          tunnel: w364 -> [w369 w373]
          frame True {
            n305 = call-poly "Enqueue Message.vi"("error in (no error)"=w369, "Message"="Confirm Quit", "Message Queue"=w370) -> ("error out"=w371:errorcluster)  [unwired: 7 in, 1 out]
          }
          frame False {
            n306 = call-poly "Enqueue Message.vi"("error in (no error)"=w373, "Message"="Load Main", "Message Queue"=w374) -> ("error out"=w375:errorcluster)  [unwired: 7 in, 1 out]
          }
        }
      }
      frame "Error" {
        # "#CodeRecommended - If you ever change the name of this \"Error\" message, you'll need to update the name in the Check Loop Error.vi as well."
        # "#CodeRecommended - Consider creating a system for logging errors in some way. These errors are for notification purposes only. Handling of specific errors should be performed in the message frames that generated the error."
        # "Error - Display an error dialog. This message is sent by the \"Error Handler\" VIs at the end of other loops in this application."
        n307 = Variant To Data(error in=w383, type=errorcluster {"status"=FALSE, "code"=0, "source"=""} ("error constant"), Variant=w381) -> (data=w379:errorcluster, error out=w378:errorcluster)
        n308 = call <vilib>:"Simple Error Handler.vi"("error in (no error)"=w379) -> ()  [unwired: 4 in, 5 out]
        n309 = Merge Errors(w378) -> (w377:errorcluster)
      }
      frame "Confirm Quit" {
        # "#CodeNeeded - If you want to provide an \"Are you sure\" dialog (or some other notification) before the application exits, place that code here. This message is typically sent from a Panel Close? event."
        # "Confirm Quit - Message that can confirm whether or not the user wants to exit the application."
        n310 = call-poly "Enqueue Message.vi"("Priority Message? (F)"=TRUE, "error in (no error)"=w390, "Message"="Exit", "Message Queue"=w386) -> ("error out"=w387:errorcluster)  [unwired: 6 in, 1 out]
        n311 = Merge Errors(w387) -> (w388:errorcluster)
      }
      frame "Exit" {
        # "Stop the VI"
        # "Release the message queue reference"
        # "#CodeNeeded - Add any required cleanup code here. Note that if 'Exit' was called as a result of an error, an error dialog will be displayed. Add any custom error handling for an 'Exit' condition here as well."
        # "Exit - Exit the application."
        n312 = call "Fire User Event - Stop.vi"("User Event - Stop"=w391) -> ("error out"=w393:errorcluster)  [unwired: 10 in]
        n313 = Release Queue(queue=w398, error in (no error)=w392) -> (error out=w395:errorcluster)  [unwired: 1 in, 2 out]
        n314 = Merge Errors(w393, w395) -> (w394:errorcluster)
      }
      frame Default {
        # "'Default' case only runs if there is a message that isn't defined in any of the other cases.  Output a programming error."
        n315 = xnode "Error Ring"("parameter 0"=w399) -> ("error out"=w400:errorcluster)
      }
    }
    n316 = call "LAB-IQ Error Handler - Message Handling Loop.vi"("error in (no error)"=w347, "Message Queue"=w349) -> ("dup error in"=w348:errorcluster)  [unwired: 8 in, 1 out]
  }
  n317 = while {
    shift-right: [w419] -> _
    shift-left: w6 -> [w420]
    tunnel: [w413] -> w15
    tunnel: w16 -> [w411]
    tunnel: w4 -> [w410]
    tunnel: w5 -> [w409]
    stop <- w418 stop-if-true
    # "Sway Motor  Handling Loop"
    n318 = call "Dequeue Message.vi"("error in (no error)"=w410, "Message Queue"=w411) -> ("error out"=w417:errorcluster, "Message Data"=w415:variant, "Message"=w416:string, "dup Message Queue"=w414:refnum<queue>)  [unwired: 6 in]
    n319 = case "Message Cases" shown="\"Exit\"" w416 {
      selector: w416 -> [_ _ _ _ _ w464]
      tunnel: w414 -> [w421 w432 _ w451 w463 _]
      tunnel: w417 -> [w424 w429 w448 w455 w457 _]
      tunnel: [w425 w433 w442 w453 w459 w465] -> w412
      tunnel: w420 -> [w423 w431 w447 w454 w462 w466]
      tunnel: [w423 w431 w447 w454 w462 w466] -> w419
      tunnel: [_ _ _ _ TRUE _] -> w418
      tunnel: w415 -> [_ _ w446 _ _ _]
      tunnel: w409 -> [_ _ _ _ w456 _]
      frame "init" {
        # "Bundle control references and a sample string value."
        # "Initialize - All initialization work should take place in this message, since other loops can potentially enqueue messages that execute immediately after this one."
        n320 = call-poly "Enqueue Message.vi"("error in (no error)"=w424, "Message"="Sway Main", "Message Queue"=w421) -> ("error out"=w425:errorcluster)  [unwired: 7 in, 1 out]
      }
      frame "Sway Main" {
        n321 = Unbundle By Name(w431) -> ("Main Home Screen.EXIT"=w430:refnum<vi>)
        n322 = property class="Bool (strict)"(reference=w430) -> (reference out=w427:refnum<vi>, error out=w428:errorcluster, "Value"=w426:bool)  [unwired: 1 in]
        n323 = Close Reference(reference=w427, error in (no error)=w428) -> ()  [unwired: 1 out]
        n324 = case shown="False" w426 {
          tunnel: [w436 w440] -> w433
          tunnel: w432 -> [w435 w439]
          tunnel: w429 -> [w434 w438]
          frame True {
            n325 = call-poly "Enqueue Message.vi"("error in (no error)"=w434, "Message"="Confirm Quit", "Message Queue"=w435) -> ("error out"=w436:errorcluster)  [unwired: 7 in, 1 out]
          }
          frame False {
            n326 = call-poly "Enqueue Message.vi"("error in (no error)"=w438, "Message"="Sway Main", "Message Queue"=w439) -> ("error out"=w440:errorcluster)  [unwired: 7 in, 1 out]
          }
        }
      }
      frame "Error" {
        # "#CodeRecommended - If you ever change the name of this \"Error\" message, you'll need to update the name in the Check Loop Error.vi as well."
        # "#CodeRecommended - Consider creating a system for logging errors in some way. These errors are for notification purposes only. Handling of specific errors should be performed in the message frames that generated the error."
        # "Error - Display an error dialog. This message is sent by the \"Error Handler\" VIs at the end of other loops in this application."
        n327 = Variant To Data(error in=w448, type=errorcluster {"status"=FALSE, "code"=0, "source"=""} ("error constant"), Variant=w446) -> (data=w444:errorcluster, error out=w443:errorcluster)
        n328 = call <vilib>:"Simple Error Handler.vi"("error in (no error)"=w444) -> ()  [unwired: 4 in, 5 out]
        n329 = Merge Errors(w443) -> (w442:errorcluster)
      }
      frame "Confirm Quit" {
        # "#CodeNeeded - If you want to provide an \"Are you sure\" dialog (or some other notification) before the application exits, place that code here. This message is typically sent from a Panel Close? event."
        # "Confirm Quit - Message that can confirm whether or not the user wants to exit the application."
        n330 = call-poly "Enqueue Message.vi"("Priority Message? (F)"=TRUE, "error in (no error)"=w455, "Message"="Exit", "Message Queue"=w451) -> ("error out"=w452:errorcluster)  [unwired: 6 in, 1 out]
        n331 = Merge Errors(w452) -> (w453:errorcluster)
      }
      frame "Exit" {
        # "Stop the VI"
        # "Release the message queue reference"
        # "#CodeNeeded - Add any required cleanup code here. Note that if 'Exit' was called as a result of an error, an error dialog will be displayed. Add any custom error handling for an 'Exit' condition here as well."
        # "Exit - Exit the application."
        n332 = call "Fire User Event - Stop.vi"("User Event - Stop"=w456) -> ("error out"=w458:errorcluster)  [unwired: 10 in]
        n333 = Release Queue(queue=w463, error in (no error)=w457) -> (error out=w460:errorcluster)  [unwired: 1 in, 2 out]
        n334 = Merge Errors(w458, w460) -> (w459:errorcluster)
      }
      frame Default {
        # "'Default' case only runs if there is a message that isn't defined in any of the other cases.  Output a programming error."
        n335 = xnode "Error Ring"("parameter 0"=w464) -> ("error out"=w465:errorcluster)
      }
    }
    n336 = call "LAB-IQ Error Handler - Message Handling Loop.vi"("error in (no error)"=w412, "Message Queue"=w414) -> ("dup error in"=w413:errorcluster)  [unwired: 8 in, 1 out]
  }
  n337 = while {
    shift-right: [w484] -> _
    shift-left: w6 -> [w485]
    tunnel: [w478] -> w12
    tunnel: w14 -> [w476]
    tunnel: w4 -> [w475]
    tunnel: w5 -> [w474]
    stop <- w483 stop-if-true
    # "Heave Motor  Handling Loop"
    n338 = call "Dequeue Message.vi"("error in (no error)"=w475, "Message Queue"=w476) -> ("error out"=w482:errorcluster, "Message Data"=w480:variant, "Message"=w481:string, "dup Message Queue"=w479:refnum<queue>)  [unwired: 6 in]
    n339 = case "Message Cases" shown="\"Exit\"" w481 {
      selector: w481 -> [_ _ _ _ _ w529]
      tunnel: w479 -> [w486 w497 _ w516 w528 _]
      tunnel: w482 -> [w489 w494 w513 w520 w522 _]
      tunnel: [w490 w498 w507 w518 w524 w530] -> w477
      tunnel: w485 -> [w488 w496 w512 w519 w527 w531]
      tunnel: [w488 w496 w512 w519 w527 w531] -> w484
      tunnel: [_ _ _ _ TRUE _] -> w483
      tunnel: w480 -> [_ _ w511 _ _ _]
      tunnel: w474 -> [_ _ _ _ w521 _]
      frame "init" {
        # "Initialize - All initialization work should take place in this message, since other loops can potentially enqueue messages that execute immediately after this one."
        n340 = call-poly "Enqueue Message.vi"("error in (no error)"=w489, "Message"="Heave Main", "Message Queue"=w486) -> ("error out"=w490:errorcluster)  [unwired: 7 in, 1 out]
      }
      frame "Heave Main" {
        n341 = Unbundle By Name(w496) -> ("Main Home Screen.EXIT"=w495:refnum<vi>)
        n342 = property class="Bool (strict)"(reference=w495) -> (reference out=w492:refnum<vi>, error out=w493:errorcluster, "Value"=w491:bool)  [unwired: 1 in]
        n343 = Close Reference(reference=w492, error in (no error)=w493) -> ()  [unwired: 1 out]
        n344 = case shown="False" w491 {
          tunnel: [w501 w505] -> w498
          tunnel: w497 -> [w500 w504]
          tunnel: w494 -> [w499 w503]
          frame True {
            n345 = call-poly "Enqueue Message.vi"("error in (no error)"=w499, "Message"="Confirm Quit", "Message Queue"=w500) -> ("error out"=w501:errorcluster)  [unwired: 7 in, 1 out]
          }
          frame False {
            n346 = call-poly "Enqueue Message.vi"("error in (no error)"=w503, "Message"="Heave Main", "Message Queue"=w504) -> ("error out"=w505:errorcluster)  [unwired: 7 in, 1 out]
          }
        }
      }
      frame "Error" {
        # "#CodeRecommended - If you ever change the name of this \"Error\" message, you'll need to update the name in the Check Loop Error.vi as well."
        # "#CodeRecommended - Consider creating a system for logging errors in some way. These errors are for notification purposes only. Handling of specific errors should be performed in the message frames that generated the error."
        # "Error - Display an error dialog. This message is sent by the \"Error Handler\" VIs at the end of other loops in this application."
        n347 = Variant To Data(error in=w513, type=errorcluster {"status"=FALSE, "code"=0, "source"=""} ("error constant"), Variant=w511) -> (data=w509:errorcluster, error out=w508:errorcluster)
        n348 = call <vilib>:"Simple Error Handler.vi"("error in (no error)"=w509) -> ()  [unwired: 4 in, 5 out]
        n349 = Merge Errors(w508) -> (w507:errorcluster)
      }
      frame "Confirm Quit" {
        # "#CodeNeeded - If you want to provide an \"Are you sure\" dialog (or some other notification) before the application exits, place that code here. This message is typically sent from a Panel Close? event."
        # "Confirm Quit - Message that can confirm whether or not the user wants to exit the application."
        n350 = call-poly "Enqueue Message.vi"("Priority Message? (F)"=TRUE, "error in (no error)"=w520, "Message"="Exit", "Message Queue"=w516) -> ("error out"=w517:errorcluster)  [unwired: 6 in, 1 out]
        n351 = Merge Errors(w517) -> (w518:errorcluster)
      }
      frame "Exit" {
        # "Stop the VI"
        # "Release the message queue reference"
        # "#CodeNeeded - Add any required cleanup code here. Note that if 'Exit' was called as a result of an error, an error dialog will be displayed. Add any custom error handling for an 'Exit' condition here as well."
        # "Exit - Exit the application."
        n352 = call "Fire User Event - Stop.vi"("User Event - Stop"=w521) -> ("error out"=w523:errorcluster)  [unwired: 10 in]
        n353 = Release Queue(queue=w528, error in (no error)=w522) -> (error out=w525:errorcluster)  [unwired: 1 in, 2 out]
        n354 = Merge Errors(w523, w525) -> (w524:errorcluster)
      }
      frame Default {
        # "'Default' case only runs if there is a message that isn't defined in any of the other cases.  Output a programming error."
        n355 = xnode "Error Ring"("parameter 0"=w529) -> ("error out"=w530:errorcluster)
      }
    }
    n356 = call "LAB-IQ Error Handler - Message Handling Loop.vi"("error in (no error)"=w477, "Message Queue"=w479) -> ("dup error in"=w478:errorcluster)  [unwired: 8 in, 1 out]
  }
  n357 = while {
    shift-right: [w549] -> _
    shift-left: w6 -> [w550]
    tunnel: [w543] -> w11
    tunnel: w13 -> [w541]
    tunnel: w4 -> [w540]
    tunnel: w5 -> [w539]
    stop <- w548 stop-if-true
    # "Temperature  Handling Loop"
    n358 = call "Dequeue Message.vi"("error in (no error)"=w540, "Message Queue"=w541) -> ("error out"=w547:errorcluster, "Message Data"=w545:variant, "Message"=w546:string, "dup Message Queue"=w544:refnum<queue>)  [unwired: 6 in]
    n359 = case "Message Cases" shown="\"Temperature Main\"" w546 {
      selector: w546 -> [_ _ _ _ _ w594]
      tunnel: w544 -> [w551 w562 _ w581 w593 _]
      tunnel: w547 -> [w554 w559 w578 w585 w587 _]
      tunnel: [w555 w563 w572 w583 w589 w595] -> w542
      tunnel: w550 -> [w553 w561 w577 w584 w592 w596]
      tunnel: [w553 w561 w577 w584 w592 w596] -> w549
      tunnel: [_ _ _ _ TRUE _] -> w548
      tunnel: w545 -> [_ _ w576 _ _ _]
      tunnel: w539 -> [_ _ _ _ w586 _]
      frame "init" {
        # "Initialize - All initialization work should take place in this message, since other loops can potentially enqueue messages that execute immediately after this one."
        n360 = call-poly "Enqueue Message.vi"("error in (no error)"=w554, "Message"="Temperature Main", "Message Queue"=w551) -> ("error out"=w555:errorcluster)  [unwired: 7 in, 1 out]
      }
      frame "Temperature Main" {
        n361 = Unbundle By Name(w561) -> ("Main Home Screen.EXIT"=w560:refnum<vi>)
        n362 = property class="Bool (strict)"(reference=w560) -> (reference out=w557:refnum<vi>, error out=w558:errorcluster, "Value"=w556:bool)  [unwired: 1 in]
        n363 = case shown="False" w556 {
          tunnel: [w566 w570] -> w563
          tunnel: w562 -> [w565 w569]
          tunnel: w559 -> [w564 w568]
          frame True {
            n364 = call-poly "Enqueue Message.vi"("error in (no error)"=w564, "Message"="Confirm Quit", "Message Queue"=w565) -> ("error out"=w566:errorcluster)  [unwired: 7 in, 1 out]
          }
          frame False {
            n365 = call-poly "Enqueue Message.vi"("error in (no error)"=w568, "Message"="Temperature Main", "Message Queue"=w569) -> ("error out"=w570:errorcluster)  [unwired: 7 in, 1 out]
          }
        }
        n366 = Close Reference(reference=w557, error in (no error)=w558) -> ()  [unwired: 1 out]
      }
      frame "Error" {
        # "#CodeRecommended - If you ever change the name of this \"Error\" message, you'll need to update the name in the Check Loop Error.vi as well."
        # "#CodeRecommended - Consider creating a system for logging errors in some way. These errors are for notification purposes only. Handling of specific errors should be performed in the message frames that generated the error."
        # "Error - Display an error dialog. This message is sent by the \"Error Handler\" VIs at the end of other loops in this application."
        n367 = Variant To Data(error in=w578, type=errorcluster {"status"=FALSE, "code"=0, "source"=""} ("error constant"), Variant=w576) -> (data=w574:errorcluster, error out=w573:errorcluster)
        n368 = call <vilib>:"Simple Error Handler.vi"("error in (no error)"=w574) -> ()  [unwired: 4 in, 5 out]
        n369 = Merge Errors(w573) -> (w572:errorcluster)
      }
      frame "Confirm Quit" {
        # "#CodeNeeded - If you want to provide an \"Are you sure\" dialog (or some other notification) before the application exits, place that code here. This message is typically sent from a Panel Close? event."
        # "Confirm Quit - Message that can confirm whether or not the user wants to exit the application."
        n370 = call-poly "Enqueue Message.vi"("Priority Message? (F)"=TRUE, "error in (no error)"=w585, "Message"="Exit", "Message Queue"=w581) -> ("error out"=w582:errorcluster)  [unwired: 6 in, 1 out]
        n371 = Merge Errors(w582) -> (w583:errorcluster)
      }
      frame "Exit" {
        # "Stop the VI"
        # "Release the message queue reference"
        # "#CodeNeeded - Add any required cleanup code here. Note that if 'Exit' was called as a result of an error, an error dialog will be displayed. Add any custom error handling for an 'Exit' condition here as well."
        # "Exit - Exit the application."
        n372 = call "Fire User Event - Stop.vi"("User Event - Stop"=w586) -> ("error out"=w588:errorcluster)  [unwired: 10 in]
        n373 = Release Queue(queue=w593, error in (no error)=w587) -> (error out=w590:errorcluster)  [unwired: 1 in, 2 out]
        n374 = Merge Errors(w588, w590) -> (w589:errorcluster)
      }
      frame Default {
        # "'Default' case only runs if there is a message that isn't defined in any of the other cases.  Output a programming error."
        n375 = xnode "Error Ring"("parameter 0"=w594) -> ("error out"=w595:errorcluster)
      }
    }
    n376 = call "LAB-IQ Error Handler - Message Handling Loop.vi"("error in (no error)"=w542, "Message Queue"=w544) -> ("dup error in"=w543:errorcluster)  [unwired: 8 in, 1 out]
  }
  n377 = while {
    shift-right: [w614] -> _
    shift-left: w6 -> [w615]
    tunnel: [w608] -> _
    tunnel: w10 -> [w606]
    tunnel: w4 -> [w605]
    tunnel: w5 -> [w604]
    stop <- w613 stop-if-true
    # "Ramp Motor  Handling Loop"
    n378 = call "Dequeue Message.vi"("error in (no error)"=w605, "Message Queue"=w606) -> ("error out"=w612:errorcluster, "Message Data"=w610:variant, "Message"=w611:string, "dup Message Queue"=w609:refnum<queue>)  [unwired: 6 in]
    n379 = case "Message Cases" shown="\"init\"" w611 {
      selector: w611 -> [_ _ _ _ _ w659]
      tunnel: w609 -> [w616 w627 _ w646 w658 _]
      tunnel: w612 -> [w619 w624 w643 w650 w652 _]
      tunnel: [w620 w628 w637 w648 w654 w660] -> w607
      tunnel: w615 -> [w618 w626 w642 w649 w657 w661]
      tunnel: [w618 w626 w642 w649 w657 w661] -> w614
      tunnel: [_ _ _ _ TRUE _] -> w613
      tunnel: w610 -> [_ _ w641 _ _ _]
      tunnel: w604 -> [_ _ _ _ w651 _]
      frame "init" {
        # "Initialize - All initialization work should take place in this message, since other loops can potentially enqueue messages that execute immediately after this one."
        n380 = call-poly "Enqueue Message.vi"("error in (no error)"=w619, "Message"="Ramp Main", "Message Queue"=w616) -> ("error out"=w620:errorcluster)  [unwired: 7 in, 1 out]
      }
      frame "Ramp Main" {
        n381 = Unbundle By Name(w626) -> ("Main Home Screen.EXIT"=w625:refnum<vi>)
        n382 = property class="Bool (strict)"(reference=w625) -> (reference out=w622:refnum<vi>, error out=w623:errorcluster, "Value"=w621:bool)  [unwired: 1 in]
        n383 = case shown="False" w621 {
          tunnel: [w631 w635] -> w628
          tunnel: w627 -> [w630 w634]
          tunnel: w624 -> [w629 w633]
          frame True {
            n384 = call-poly "Enqueue Message.vi"("error in (no error)"=w629, "Message"="Confirm Quit", "Message Queue"=w630) -> ("error out"=w631:errorcluster)  [unwired: 7 in, 1 out]
          }
          frame False {
            n385 = call-poly "Enqueue Message.vi"("error in (no error)"=w633, "Message"="Ramp Main", "Message Queue"=w634) -> ("error out"=w635:errorcluster)  [unwired: 7 in, 1 out]
          }
        }
        n386 = Close Reference(reference=w622, error in (no error)=w623) -> ()  [unwired: 1 out]
      }
      frame "Error" {
        # "#CodeRecommended - If you ever change the name of this \"Error\" message, you'll need to update the name in the Check Loop Error.vi as well."
        # "#CodeRecommended - Consider creating a system for logging errors in some way. These errors are for notification purposes only. Handling of specific errors should be performed in the message frames that generated the error."
        # "Error - Display an error dialog. This message is sent by the \"Error Handler\" VIs at the end of other loops in this application."
        n387 = Variant To Data(error in=w643, type=errorcluster {"status"=FALSE, "code"=0, "source"=""} ("error constant"), Variant=w641) -> (data=w639:errorcluster, error out=w638:errorcluster)
        n388 = call <vilib>:"Simple Error Handler.vi"("error in (no error)"=w639) -> ()  [unwired: 4 in, 5 out]
        n389 = Merge Errors(w638) -> (w637:errorcluster)
      }
      frame "Confirm Quit" {
        # "#CodeNeeded - If you want to provide an \"Are you sure\" dialog (or some other notification) before the application exits, place that code here. This message is typically sent from a Panel Close? event."
        # "Confirm Quit - Message that can confirm whether or not the user wants to exit the application."
        n390 = call-poly "Enqueue Message.vi"("Priority Message? (F)"=TRUE, "error in (no error)"=w650, "Message"="Exit", "Message Queue"=w646) -> ("error out"=w647:errorcluster)  [unwired: 6 in, 1 out]
        n391 = Merge Errors(w647) -> (w648:errorcluster)
      }
      frame "Exit" {
        # "Stop the VI"
        # "Release the message queue reference"
        # "#CodeNeeded - Add any required cleanup code here. Note that if 'Exit' was called as a result of an error, an error dialog will be displayed. Add any custom error handling for an 'Exit' condition here as well."
        # "Exit - Exit the application."
        n392 = call "Fire User Event - Stop.vi"("User Event - Stop"=w651) -> ("error out"=w653:errorcluster)  [unwired: 10 in]
        n393 = Release Queue(queue=w658, error in (no error)=w652) -> (error out=w655:errorcluster)  [unwired: 1 in, 2 out]
        n394 = Merge Errors(w653, w655) -> (w654:errorcluster)
      }
      frame Default {
        # "'Default' case only runs if there is a message that isn't defined in any of the other cases.  Output a programming error."
        n395 = xnode "Error Ring"("parameter 0"=w659) -> ("error out"=w660:errorcluster)
      }
    }
    n396 = call "LAB-IQ Error Handler - Message Handling Loop.vi"("error in (no error)"=w607, "Message Queue"=w609) -> ("dup error in"=w608:errorcluster)  [unwired: 8 in, 1 out]
  }
  n397 = while {
    shift-right: [w679] -> _
    shift-left: w6 -> [w680]
    tunnel: [w673] -> _
    tunnel: w9 -> [w671]
    tunnel: w4 -> [w670]
    tunnel: w5 -> [w669]
    stop <- w678 stop-if-true
    # "ECR  Handling Loop"
    n398 = call "Dequeue Message.vi"("error in (no error)"=w670, "Message Queue"=w671) -> ("error out"=w677:errorcluster, "Message Data"=w675:variant, "Message"=w676:string, "dup Message Queue"=w674:refnum<queue>)  [unwired: 6 in]
    n399 = case "Message Cases" shown="\"ECR Main\"" w676 {
      selector: w676 -> [_ _ _ _ _ w724]
      tunnel: w674 -> [w681 w692 _ w711 w723 _]
      tunnel: w677 -> [w684 w689 w708 w715 w717 _]
      tunnel: [w685 w693 w702 w713 w719 w725] -> w672
      tunnel: w680 -> [w683 w691 w707 w714 w722 w726]
      tunnel: [w683 w691 w707 w714 w722 w726] -> w679
      tunnel: [_ _ _ _ TRUE _] -> w678
      tunnel: w675 -> [_ _ w706 _ _ _]
      tunnel: w669 -> [_ _ _ _ w716 _]
      frame "init" {
        # "Initialize - All initialization work should take place in this message, since other loops can potentially enqueue messages that execute immediately after this one."
        n400 = call-poly "Enqueue Message.vi"("error in (no error)"=w684, "Message"="ECR Main", "Message Queue"=w681) -> ("error out"=w685:errorcluster)  [unwired: 7 in, 1 out]
      }
      frame "ECR Main" {
        n401 = Unbundle By Name(w691) -> ("Main Home Screen.EXIT"=w690:refnum<vi>)
        n402 = property class="Bool (strict)"(reference=w690) -> (reference out=w687:refnum<vi>, error out=w688:errorcluster, "Value"=w686:bool)  [unwired: 1 in]
        n403 = case shown="False" w686 {
          tunnel: [w696 w700] -> w693
          tunnel: w692 -> [w695 w699]
          tunnel: w689 -> [w694 w698]
          frame True {
            n404 = call-poly "Enqueue Message.vi"("error in (no error)"=w694, "Message"="Confirm Quit", "Message Queue"=w695) -> ("error out"=w696:errorcluster)  [unwired: 7 in, 1 out]
          }
          frame False {
            n405 = call-poly "Enqueue Message.vi"("error in (no error)"=w698, "Message"="ECR Main", "Message Queue"=w699) -> ("error out"=w700:errorcluster)  [unwired: 7 in, 1 out]
          }
        }
        n406 = Close Reference(reference=w687, error in (no error)=w688) -> ()  [unwired: 1 out]
      }
      frame "Error" {
        # "#CodeRecommended - If you ever change the name of this \"Error\" message, you'll need to update the name in the Check Loop Error.vi as well."
        # "#CodeRecommended - Consider creating a system for logging errors in some way. These errors are for notification purposes only. Handling of specific errors should be performed in the message frames that generated the error."
        # "Error - Display an error dialog. This message is sent by the \"Error Handler\" VIs at the end of other loops in this application."
        n407 = Variant To Data(error in=w708, type=errorcluster {"status"=FALSE, "code"=0, "source"=""} ("error constant"), Variant=w706) -> (data=w704:errorcluster, error out=w703:errorcluster)
        n408 = call <vilib>:"Simple Error Handler.vi"("error in (no error)"=w704) -> ()  [unwired: 4 in, 5 out]
        n409 = Merge Errors(w703) -> (w702:errorcluster)
      }
      frame "Confirm Quit" {
        # "#CodeNeeded - If you want to provide an \"Are you sure\" dialog (or some other notification) before the application exits, place that code here. This message is typically sent from a Panel Close? event."
        # "Confirm Quit - Message that can confirm whether or not the user wants to exit the application."
        n410 = call-poly "Enqueue Message.vi"("Priority Message? (F)"=TRUE, "error in (no error)"=w715, "Message"="Exit", "Message Queue"=w711) -> ("error out"=w712:errorcluster)  [unwired: 6 in, 1 out]
        n411 = Merge Errors(w712) -> (w713:errorcluster)
      }
      frame "Exit" {
        # "Stop the VI"
        # "Release the message queue reference"
        # "#CodeNeeded - Add any required cleanup code here. Note that if 'Exit' was called as a result of an error, an error dialog will be displayed. Add any custom error handling for an 'Exit' condition here as well."
        # "Exit - Exit the application."
        n412 = call "Fire User Event - Stop.vi"("User Event - Stop"=w716) -> ("error out"=w718:errorcluster)  [unwired: 10 in]
        n413 = Release Queue(queue=w723, error in (no error)=w717) -> (error out=w720:errorcluster)  [unwired: 1 in, 2 out]
        n414 = Merge Errors(w718, w720) -> (w719:errorcluster)
      }
      frame Default {
        # "'Default' case only runs if there is a message that isn't defined in any of the other cases.  Output a programming error."
        n415 = xnode "Error Ring"("parameter 0"=w724) -> ("error out"=w725:errorcluster)
      }
    }
    n416 = call "LAB-IQ Error Handler - Message Handling Loop.vi"("error in (no error)"=w672, "Message Queue"=w674) -> ("dup error in"=w673:errorcluster)  [unwired: 8 in, 1 out]
  }
  n417 = while {
    tunnel: w45 -> [w748]
    shift-right: [w755] -> _
    shift-left: w6 -> [w756]
    tunnel: w5 -> [w753]
    tunnel: w38 -> [w752]
    tunnel: [w746] -> w46
    tunnel: w17 -> [w744]
    tunnel: w16 -> [w743]
    tunnel: w14 -> [w742]
    tunnel: w13 -> [w741]
    tunnel: w10 -> [w740]
    tunnel: w9 -> [w739]
    tunnel: w8 -> [w738]
    tunnel: w7 -> [w737]
    tunnel: w3 -> [w736]
    tunnel: w2 -> [w735]
    tunnel: w1 -> [w734]
    stop <- w754 stop-if-true
    # "Message Handling Loop"
    n418 = call "Dequeue Message.vi"("error in (no error)"=w752, "Message Queue"=w748) -> ("error out"=w751:errorcluster, "Message Data"=w749:variant, "Message"=w750:string, "dup Message Queue"=w747:refnum<queue>)  [unwired: 6 in]
    n419 = case "Message Cases" shown="Default" w750 {
      selector: w750 -> [_ _ _ _ _ _ w811]
      tunnel: w747 -> [_ w759 _ _ w798 w810 _]
      tunnel: w751 -> [w758 w762 w787 w795 w802 w803 _]
      tunnel: [w758 w763 w776 w789 w800 w806 w812] -> w745
      tunnel: w756 -> [w757 w761 w788 w794 w801 w809 w813]
      tunnel: [w757 w761 w788 w794 w801 w809 w813] -> w755
      tunnel: [_ _ _ _ _ TRUE _] -> w754
      tunnel: w749 -> [_ _ _ w793 _ _ _]
      tunnel: w753 -> [_ _ _ _ _ w805 _]
      tunnel: w744 -> [_ _ w774 _ _ _ _]
      tunnel: w743 -> [_ _ w773 _ _ _ _]
      tunnel: w742 -> [_ _ w772 _ _ _ _]
      tunnel: w741 -> [_ _ w771 _ _ _ _]
      tunnel: w740 -> [_ _ w770 _ _ _ _]
      tunnel: w739 -> [_ _ w769 _ _ _ _]
      tunnel: w738 -> [_ _ w768 _ _ _ _]
      tunnel: w737 -> [_ _ w767 _ _ _ _]
      tunnel: w736 -> [_ _ w766 _ _ _ _]
      tunnel: w735 -> [_ _ w765 _ _ _ _]
      tunnel: w734 -> [_ _ w764 _ _ _ _]
      frame "Time Out" {
      }
      frame "init" {
        # "Bundle control references and a sample string value."
        # "Initialize - All initialization work should take place in this message, since other loops can potentially enqueue messages that execute immediately after this one."
        n420 = call-poly "Enqueue Message.vi"("error in (no error)"=w762, "Message"="Init Other Loop", "Message Queue"=w759) -> ("error out"=w763:errorcluster)  [unwired: 7 in, 1 out]
      }
      frame "Init Other Loop" {
        w775 = "Init" ("Message")
        n421 = call-poly "Enqueue Message.vi"("error in (no error)"=w787, "Message"=w775, "Message Queue"=w774) -> ("error out"=w786:errorcluster)  [unwired: 7 in, 1 out]
        n422 = call-poly "Enqueue Message.vi"("error in (no error)"=w786, "Message"=w775, "Message Queue"=w773) -> ("error out"=w785:errorcluster)  [unwired: 7 in, 1 out]
        n423 = call-poly "Enqueue Message.vi"("error in (no error)"=w785, "Message"=w775, "Message Queue"=w772) -> ("error out"=w784:errorcluster)  [unwired: 7 in, 1 out]
        n424 = call-poly "Enqueue Message.vi"("error in (no error)"=w784, "Message"=w775, "Message Queue"=w771) -> ("error out"=w783:errorcluster)  [unwired: 7 in, 1 out]
        n425 = call-poly "Enqueue Message.vi"("error in (no error)"=w783, "Message"=w775, "Message Queue"=w770) -> ("error out"=w782:errorcluster)  [unwired: 7 in, 1 out]
        n426 = call-poly "Enqueue Message.vi"("error in (no error)"=w782, "Message"=w775, "Message Queue"=w769) -> ("error out"=w781:errorcluster)  [unwired: 7 in, 1 out]
        n427 = call-poly "Enqueue Message.vi"("error in (no error)"=w781, "Message"=w775, "Message Queue"=w768) -> ("error out"=w780:errorcluster)  [unwired: 7 in, 1 out]
        n428 = call-poly "Enqueue Message.vi"("error in (no error)"=w780, "Message"=w775, "Message Queue"=w767) -> ("error out"=w779:errorcluster)  [unwired: 7 in, 1 out]
        n429 = call-poly "Enqueue Message.vi"("error in (no error)"=w779, "Message"=w775, "Message Queue"=w766) -> ("error out"=w778:errorcluster)  [unwired: 7 in, 1 out]
        n430 = call-poly "Enqueue Message.vi"("error in (no error)"=w778, "Message"=w775, "Message Queue"=w765) -> ("error out"=w777:errorcluster)  [unwired: 7 in, 1 out]
        n431 = call-poly "Enqueue Message.vi"("error in (no error)"=w777, "Message"=w775, "Message Queue"=w764) -> ("error out"=w776:errorcluster)  [unwired: 7 in, 1 out]
      }
      frame "Error" {
        # "#CodeRecommended - If you ever change the name of this \"Error\" message, you'll need to update the name in the Check Loop Error.vi as well."
        # "#CodeRecommended - Consider creating a system for logging errors in some way. These errors are for notification purposes only. Handling of specific errors should be performed in the message frames that generated the error."
        # "Error - Display an error dialog. This message is sent by the \"Error Handler\" VIs at the end of other loops in this application."
        n432 = Variant To Data(error in=w795, type=errorcluster {"status"=FALSE, "code"=0, "source"=""} ("error constant"), Variant=w793) -> (data=w791:errorcluster, error out=w790:errorcluster)
        n433 = call <vilib>:"Simple Error Handler.vi"("error in (no error)"=w791) -> ()  [unwired: 4 in, 5 out]
        n434 = Merge Errors(w790) -> (w789:errorcluster)
      }
      frame "Confirm Quit" {
        # "#CodeNeeded - If you want to provide an \"Are you sure\" dialog (or some other notification) before the application exits, place that code here. This message is typically sent from a Panel Close? event."
        # "Confirm Quit - Message that can confirm whether or not the user wants to exit the application."
        n435 = call-poly "Enqueue Message.vi"("Priority Message? (F)"=TRUE, "error in (no error)"=w802, "Message"="Exit", "Message Queue"=w798) -> ("error out"=w799:errorcluster)  [unwired: 6 in, 1 out]
        n436 = Merge Errors(w799) -> (w800:errorcluster)
      }
      frame "Exit" {
        # "Stop the VI"
        # "Release the message queue reference"
        # "#CodeNeeded - Add any required cleanup code here. Note that if 'Exit' was called as a result of an error, an error dialog will be displayed. Add any custom error handling for an 'Exit' condition here as well."
        # "Exit - Exit the application."
        n437 = call "Fire User Event - Stop.vi"("User Event - Stop"=w805) -> ("error out"=w804:errorcluster)  [unwired: 10 in]
        n438 = Release Queue(queue=w810, error in (no error)=w803) -> (error out=w807:errorcluster)  [unwired: 1 in, 2 out]
        n439 = Merge Errors(w804, w807) -> (w806:errorcluster)
      }
      frame Default {
        # "'Default' case only runs if there is a message that isn't defined in any of the other cases.  Output a programming error."
        n440 = xnode "Error Ring"("parameter 0"=w811) -> ("error out"=w812:errorcluster)
      }
    }
    n441 = call "LAB-IQ Error Handler - Message Handling Loop.vi"("error in (no error)"=w745, "Message Queue"=w747) -> ("dup error in"=w746:errorcluster)  [unwired: 8 in, 1 out]
  }
  n442 = while {
    shift-right: [w831] -> _
    shift-left: w6 -> [w832]
    tunnel: [w825] -> _
    tunnel: w8 -> [w823]
    tunnel: w4 -> [w822]
    tunnel: w5 -> [w821]
    stop <- w830 stop-if-true
    # "Humidity  Handling Loop"
    n443 = call "Dequeue Message.vi"("error in (no error)"=w822, "Message Queue"=w823) -> ("error out"=w829:errorcluster, "Message Data"=w827:variant, "Message"=w828:string, "dup Message Queue"=w826:refnum<queue>)  [unwired: 6 in]
    n444 = case "Message Cases" shown="\"Humidity Main\"" w828 {
      selector: w828 -> [_ _ _ _ _ w876]
      tunnel: w826 -> [w833 w844 _ w863 w875 _]
      tunnel: w829 -> [w836 w841 w860 w867 w869 _]
      tunnel: [w837 w845 w854 w865 w871 w877] -> w824
      tunnel: w832 -> [w835 w843 w859 w866 w874 w878]
      tunnel: [w835 w843 w859 w866 w874 w878] -> w831
      tunnel: [_ _ _ _ TRUE _] -> w830
      tunnel: w827 -> [_ _ w858 _ _ _]
      tunnel: w821 -> [_ _ _ _ w868 _]
      frame "init" {
        # "Initialize - All initialization work should take place in this message, since other loops can potentially enqueue messages that execute immediately after this one."
        n445 = call-poly "Enqueue Message.vi"("error in (no error)"=w836, "Message"="Humidity Main", "Message Queue"=w833) -> ("error out"=w837:errorcluster)  [unwired: 7 in, 1 out]
      }
      frame "Humidity Main" {
        n446 = Unbundle By Name(w843) -> ("Main Home Screen.EXIT"=w842:refnum<vi>)
        n447 = property class="Bool (strict)"(reference=w842) -> (reference out=w839:refnum<vi>, error out=w840:errorcluster, "Value"=w838:bool)  [unwired: 1 in]
        n448 = case shown="False" w838 {
          tunnel: [w848 w852] -> w845
          tunnel: w844 -> [w847 w851]
          tunnel: w841 -> [w846 w850]
          frame True {
            n449 = call-poly "Enqueue Message.vi"("error in (no error)"=w846, "Message"="Confirm Quit", "Message Queue"=w847) -> ("error out"=w848:errorcluster)  [unwired: 7 in, 1 out]
          }
          frame False {
            n450 = call-poly "Enqueue Message.vi"("error in (no error)"=w850, "Message"="Humidity Main", "Message Queue"=w851) -> ("error out"=w852:errorcluster)  [unwired: 7 in, 1 out]
          }
        }
        n451 = Close Reference(reference=w839, error in (no error)=w840) -> ()  [unwired: 1 out]
      }
      frame "Error" {
        # "#CodeRecommended - If you ever change the name of this \"Error\" message, you'll need to update the name in the Check Loop Error.vi as well."
        # "#CodeRecommended - Consider creating a system for logging errors in some way. These errors are for notification purposes only. Handling of specific errors should be performed in the message frames that generated the error."
        # "Error - Display an error dialog. This message is sent by the \"Error Handler\" VIs at the end of other loops in this application."
        n452 = Variant To Data(error in=w860, type=errorcluster {"status"=FALSE, "code"=0, "source"=""} ("error constant"), Variant=w858) -> (data=w856:errorcluster, error out=w855:errorcluster)
        n453 = call <vilib>:"Simple Error Handler.vi"("error in (no error)"=w856) -> ()  [unwired: 4 in, 5 out]
        n454 = Merge Errors(w855) -> (w854:errorcluster)
      }
      frame "Confirm Quit" {
        # "#CodeNeeded - If you want to provide an \"Are you sure\" dialog (or some other notification) before the application exits, place that code here. This message is typically sent from a Panel Close? event."
        # "Confirm Quit - Message that can confirm whether or not the user wants to exit the application."
        n455 = call-poly "Enqueue Message.vi"("Priority Message? (F)"=TRUE, "error in (no error)"=w867, "Message"="Exit", "Message Queue"=w863) -> ("error out"=w864:errorcluster)  [unwired: 6 in, 1 out]
        n456 = Merge Errors(w864) -> (w865:errorcluster)
      }
      frame "Exit" {
        # "Stop the VI"
        # "Release the message queue reference"
        # "#CodeNeeded - Add any required cleanup code here. Note that if 'Exit' was called as a result of an error, an error dialog will be displayed. Add any custom error handling for an 'Exit' condition here as well."
        # "Exit - Exit the application."
        n457 = call "Fire User Event - Stop.vi"("User Event - Stop"=w868) -> ("error out"=w870:errorcluster)  [unwired: 10 in]
        n458 = Release Queue(queue=w875, error in (no error)=w869) -> (error out=w872:errorcluster)  [unwired: 1 in, 2 out]
        n459 = Merge Errors(w870, w872) -> (w871:errorcluster)
      }
      frame Default {
        # "'Default' case only runs if there is a message that isn't defined in any of the other cases.  Output a programming error."
        n460 = xnode "Error Ring"("parameter 0"=w876) -> ("error out"=w877:errorcluster)
      }
    }
    n461 = call "LAB-IQ Error Handler - Message Handling Loop.vi"("error in (no error)"=w824, "Message Queue"=w826) -> ("dup error in"=w825:errorcluster)  [unwired: 8 in, 1 out]
  }
  n462 = while {
    shift-right: [w896] -> _
    shift-left: w6 -> [w897]
    tunnel: [w890] -> _
    tunnel: w7 -> [w888]
    tunnel: w4 -> [w887]
    tunnel: w5 -> [w886]
    stop <- w895 stop-if-true
    # "Program  Handling Loop"
    n463 = call "Dequeue Message.vi"("error in (no error)"=w887, "Message Queue"=w888) -> ("error out"=w894:errorcluster, "Message Data"=w892:variant, "Message"=w893:string, "dup Message Queue"=w891:refnum<queue>)  [unwired: 6 in]
    n464 = case "Message Cases" shown="Default" w893 {
      selector: w893 -> [_ _ _ _ _ w941]
      tunnel: w891 -> [w898 w909 _ w928 w940 _]
      tunnel: w894 -> [w901 w906 w925 w932 w934 _]
      tunnel: [w902 w910 w919 w930 w936 w942] -> w889
      tunnel: w897 -> [w900 w908 w924 w931 w939 w943]
      tunnel: [w900 w908 w924 w931 w939 w943] -> w896
      tunnel: [_ _ _ _ TRUE _] -> w895
      tunnel: w892 -> [_ _ w923 _ _ _]
      tunnel: w886 -> [_ _ _ _ w933 _]
      frame "init" {
        # "Initialize - All initialization work should take place in this message, since other loops can potentially enqueue messages that execute immediately after this one."
        n465 = call-poly "Enqueue Message.vi"("error in (no error)"=w901, "Message"="Program Main", "Message Queue"=w898) -> ("error out"=w902:errorcluster)  [unwired: 7 in, 1 out]
      }
      frame "Program Main" {
        n466 = Unbundle By Name(w908) -> ("Main Home Screen.EXIT"=w907:refnum<vi>)
        n467 = property class="Bool (strict)"(reference=w907) -> (reference out=w904:refnum<vi>, error out=w905:errorcluster, "Value"=w903:bool)  [unwired: 1 in]
        n468 = case shown="False" w903 {
          tunnel: [w913 w917] -> w910
          tunnel: w909 -> [w912 w916]
          tunnel: w906 -> [w911 w915]
          frame True {
            n469 = call-poly "Enqueue Message.vi"("error in (no error)"=w911, "Message"="Confirm Quit", "Message Queue"=w912) -> ("error out"=w913:errorcluster)  [unwired: 7 in, 1 out]
          }
          frame False {
            n470 = call-poly "Enqueue Message.vi"("error in (no error)"=w915, "Message"="Program Main", "Message Queue"=w916) -> ("error out"=w917:errorcluster)  [unwired: 7 in, 1 out]
          }
        }
        n471 = Close Reference(reference=w904, error in (no error)=w905) -> ()  [unwired: 1 out]
      }
      frame "Error" {
        # "#CodeRecommended - If you ever change the name of this \"Error\" message, you'll need to update the name in the Check Loop Error.vi as well."
        # "#CodeRecommended - Consider creating a system for logging errors in some way. These errors are for notification purposes only. Handling of specific errors should be performed in the message frames that generated the error."
        # "Error - Display an error dialog. This message is sent by the \"Error Handler\" VIs at the end of other loops in this application."
        n472 = Variant To Data(error in=w925, type=errorcluster {"status"=FALSE, "code"=0, "source"=""} ("error constant"), Variant=w923) -> (data=w921:errorcluster, error out=w920:errorcluster)
        n473 = call <vilib>:"Simple Error Handler.vi"("error in (no error)"=w921) -> ()  [unwired: 4 in, 5 out]
        n474 = Merge Errors(w920) -> (w919:errorcluster)
      }
      frame "Confirm Quit" {
        # "#CodeNeeded - If you want to provide an \"Are you sure\" dialog (or some other notification) before the application exits, place that code here. This message is typically sent from a Panel Close? event."
        # "Confirm Quit - Message that can confirm whether or not the user wants to exit the application."
        n475 = call-poly "Enqueue Message.vi"("Priority Message? (F)"=TRUE, "error in (no error)"=w932, "Message"="Exit", "Message Queue"=w928) -> ("error out"=w929:errorcluster)  [unwired: 6 in, 1 out]
        n476 = Merge Errors(w929) -> (w930:errorcluster)
      }
      frame "Exit" {
        # "Stop the VI"
        # "Release the message queue reference"
        # "#CodeNeeded - Add any required cleanup code here. Note that if 'Exit' was called as a result of an error, an error dialog will be displayed. Add any custom error handling for an 'Exit' condition here as well."
        # "Exit - Exit the application."
        n477 = call "Fire User Event - Stop.vi"("User Event - Stop"=w933) -> ("error out"=w935:errorcluster)  [unwired: 10 in]
        n478 = Release Queue(queue=w940, error in (no error)=w934) -> (error out=w937:errorcluster)  [unwired: 1 in, 2 out]
        n479 = Merge Errors(w935, w937) -> (w936:errorcluster)
      }
      frame Default {
        # "'Default' case only runs if there is a message that isn't defined in any of the other cases.  Output a programming error."
        n480 = xnode "Error Ring"("parameter 0"=w941) -> ("error out"=w942:errorcluster)
      }
    }
    n481 = call "LAB-IQ Error Handler - Message Handling Loop.vi"("error in (no error)"=w889, "Message Queue"=w891) -> ("dup error in"=w890:errorcluster)  [unwired: 8 in, 1 out]
  }
  n482 = while {
    shift-right: [w961] -> _
    shift-left: w6 -> [w962]
    tunnel: [w955] -> _
    tunnel: w3 -> [w953]
    tunnel: w4 -> [w952]
    tunnel: w5 -> [w951]
    stop <- w960 stop-if-true
    # "Monitor  Handling Loop"
    n483 = call "Dequeue Message.vi"("error in (no error)"=w952, "Message Queue"=w953) -> ("error out"=w959:errorcluster, "Message Data"=w957:variant, "Message"=w958:string, "dup Message Queue"=w956:refnum<queue>)  [unwired: 6 in]
    n484 = case "Message Cases" shown="\"Monitor Main\"" w958 {
      selector: w958 -> [_ _ _ _ _ w1006]
      tunnel: w956 -> [w963 w974 _ w993 w1005 _]
      tunnel: w959 -> [w966 w971 w990 w997 w999 _]
      tunnel: [w967 w975 w984 w995 w1001 w1007] -> w954
      tunnel: w962 -> [w965 w973 w989 w996 w1004 w1008]
      tunnel: [w965 w973 w989 w996 w1004 w1008] -> w961
      tunnel: [_ _ _ _ TRUE _] -> w960
      tunnel: w957 -> [_ _ w988 _ _ _]
      tunnel: w951 -> [_ _ _ _ w998 _]
      frame "init" {
        # "Initialize - All initialization work should take place in this message, since other loops can potentially enqueue messages that execute immediately after this one."
        n485 = call-poly "Enqueue Message.vi"("error in (no error)"=w966, "Message"="Monitor Main", "Message Queue"=w963) -> ("error out"=w967:errorcluster)  [unwired: 7 in, 1 out]
      }
      frame "Monitor Main" {
        n486 = Unbundle By Name(w973) -> ("Main Home Screen.EXIT"=w972:refnum<vi>)
        n487 = property class="Bool (strict)"(reference=w972) -> (reference out=w969:refnum<vi>, error out=w970:errorcluster, "Value"=w968:bool)  [unwired: 1 in]
        n488 = case shown="False" w968 {
          tunnel: [w978 w982] -> w975
          tunnel: w974 -> [w977 w981]
          tunnel: w971 -> [w976 w980]
          frame True {
            n489 = call-poly "Enqueue Message.vi"("error in (no error)"=w976, "Message"="Confirm Quit", "Message Queue"=w977) -> ("error out"=w978:errorcluster)  [unwired: 7 in, 1 out]
          }
          frame False {
            n490 = call-poly "Enqueue Message.vi"("error in (no error)"=w980, "Message"="Monitor Main", "Message Queue"=w981) -> ("error out"=w982:errorcluster)  [unwired: 7 in, 1 out]
          }
        }
        n491 = Close Reference(reference=w969, error in (no error)=w970) -> ()  [unwired: 1 out]
      }
      frame "Error" {
        # "#CodeRecommended - If you ever change the name of this \"Error\" message, you'll need to update the name in the Check Loop Error.vi as well."
        # "#CodeRecommended - Consider creating a system for logging errors in some way. These errors are for notification purposes only. Handling of specific errors should be performed in the message frames that generated the error."
        # "Error - Display an error dialog. This message is sent by the \"Error Handler\" VIs at the end of other loops in this application."
        n492 = Variant To Data(error in=w990, type=errorcluster {"status"=FALSE, "code"=0, "source"=""} ("error constant"), Variant=w988) -> (data=w986:errorcluster, error out=w985:errorcluster)
        n493 = call <vilib>:"Simple Error Handler.vi"("error in (no error)"=w986) -> ()  [unwired: 4 in, 5 out]
        n494 = Merge Errors(w985) -> (w984:errorcluster)
      }
      frame "Confirm Quit" {
        # "#CodeNeeded - If you want to provide an \"Are you sure\" dialog (or some other notification) before the application exits, place that code here. This message is typically sent from a Panel Close? event."
        # "Confirm Quit - Message that can confirm whether or not the user wants to exit the application."
        n495 = call-poly "Enqueue Message.vi"("Priority Message? (F)"=TRUE, "error in (no error)"=w997, "Message"="Exit", "Message Queue"=w993) -> ("error out"=w994:errorcluster)  [unwired: 6 in, 1 out]
        n496 = Merge Errors(w994) -> (w995:errorcluster)
      }
      frame "Exit" {
        # "Stop the VI"
        # "Release the message queue reference"
        # "#CodeNeeded - Add any required cleanup code here. Note that if 'Exit' was called as a result of an error, an error dialog will be displayed. Add any custom error handling for an 'Exit' condition here as well."
        # "Exit - Exit the application."
        n497 = call "Fire User Event - Stop.vi"("User Event - Stop"=w998) -> ("error out"=w1000:errorcluster)  [unwired: 10 in]
        n498 = Release Queue(queue=w1005, error in (no error)=w999) -> (error out=w1002:errorcluster)  [unwired: 1 in, 2 out]
        n499 = Merge Errors(w1000, w1002) -> (w1001:errorcluster)
      }
      frame Default {
        # "'Default' case only runs if there is a message that isn't defined in any of the other cases.  Output a programming error."
        n500 = xnode "Error Ring"("parameter 0"=w1006) -> ("error out"=w1007:errorcluster)
      }
    }
    n501 = call "LAB-IQ Error Handler - Message Handling Loop.vi"("error in (no error)"=w954, "Message Queue"=w956) -> ("dup error in"=w955:errorcluster)  [unwired: 8 in, 1 out]
  }
  n502 = while {
    shift-right: [w1026] -> _
    shift-left: w6 -> [w1027]
    tunnel: [w1020] -> _
    tunnel: w2 -> [w1018]
    tunnel: w4 -> [w1017]
    tunnel: w5 -> [w1016]
    stop <- w1025 stop-if-true
    # "Load Pid  Handling Loop"
    n503 = call "Dequeue Message.vi"("error in (no error)"=w1017, "Message Queue"=w1018) -> ("error out"=w1024:errorcluster, "Message Data"=w1022:variant, "Message"=w1023:string, "dup Message Queue"=w1021:refnum<queue>)  [unwired: 6 in]
    n504 = case "Message Cases" shown="\"Load Pid Main\"" w1023 {
      selector: w1023 -> [_ _ _ _ _ w1071]
      tunnel: w1021 -> [w1028 w1039 _ w1058 w1070 _]
      tunnel: w1024 -> [w1031 w1036 w1055 w1062 w1064 _]
      tunnel: [w1032 w1040 w1049 w1060 w1066 w1072] -> w1019
      tunnel: w1027 -> [w1030 w1038 w1054 w1061 w1069 w1073]
      tunnel: [w1030 w1038 w1054 w1061 w1069 w1073] -> w1026
      tunnel: [_ _ _ _ TRUE _] -> w1025
      tunnel: w1022 -> [_ _ w1053 _ _ _]
      tunnel: w1016 -> [_ _ _ _ w1063 _]
      frame "init" {
        # "Initialize - All initialization work should take place in this message, since other loops can potentially enqueue messages that execute immediately after this one."
        n505 = call-poly "Enqueue Message.vi"("error in (no error)"=w1031, "Message"="Load Pid Main", "Message Queue"=w1028) -> ("error out"=w1032:errorcluster)  [unwired: 7 in, 1 out]
      }
      frame "Load Pid Main" {
        n506 = Unbundle By Name(w1038) -> ("Main Home Screen.EXIT"=w1037:refnum<vi>)
        n507 = property class="Bool (strict)"(reference=w1037) -> (reference out=w1034:refnum<vi>, error out=w1035:errorcluster, "Value"=w1033:bool)  [unwired: 1 in]
        n508 = case shown="False" w1033 {
          tunnel: [w1043 w1047] -> w1040
          tunnel: w1039 -> [w1042 w1046]
          tunnel: w1036 -> [w1041 w1045]
          frame True {
            n509 = call-poly "Enqueue Message.vi"("error in (no error)"=w1041, "Message"="Confirm Quit", "Message Queue"=w1042) -> ("error out"=w1043:errorcluster)  [unwired: 7 in, 1 out]
          }
          frame False {
            n510 = call-poly "Enqueue Message.vi"("error in (no error)"=w1045, "Message"="Load Pid Main", "Message Queue"=w1046) -> ("error out"=w1047:errorcluster)  [unwired: 7 in, 1 out]
          }
        }
        n511 = Close Reference(reference=w1034, error in (no error)=w1035) -> ()  [unwired: 1 out]
      }
      frame "Error" {
        # "#CodeRecommended - If you ever change the name of this \"Error\" message, you'll need to update the name in the Check Loop Error.vi as well."
        # "#CodeRecommended - Consider creating a system for logging errors in some way. These errors are for notification purposes only. Handling of specific errors should be performed in the message frames that generated the error."
        # "Error - Display an error dialog. This message is sent by the \"Error Handler\" VIs at the end of other loops in this application."
        n512 = Variant To Data(error in=w1055, type=errorcluster {"status"=FALSE, "code"=0, "source"=""} ("error constant"), Variant=w1053) -> (data=w1051:errorcluster, error out=w1050:errorcluster)
        n513 = call <vilib>:"Simple Error Handler.vi"("error in (no error)"=w1051) -> ()  [unwired: 4 in, 5 out]
        n514 = Merge Errors(w1050) -> (w1049:errorcluster)
      }
      frame "Confirm Quit" {
        # "#CodeNeeded - If you want to provide an \"Are you sure\" dialog (or some other notification) before the application exits, place that code here. This message is typically sent from a Panel Close? event."
        # "Confirm Quit - Message that can confirm whether or not the user wants to exit the application."
        n515 = call-poly "Enqueue Message.vi"("Priority Message? (F)"=TRUE, "error in (no error)"=w1062, "Message"="Exit", "Message Queue"=w1058) -> ("error out"=w1059:errorcluster)  [unwired: 6 in, 1 out]
        n516 = Merge Errors(w1059) -> (w1060:errorcluster)
      }
      frame "Exit" {
        # "Stop the VI"
        # "Release the message queue reference"
        # "#CodeNeeded - Add any required cleanup code here. Note that if 'Exit' was called as a result of an error, an error dialog will be displayed. Add any custom error handling for an 'Exit' condition here as well."
        # "Exit - Exit the application."
        n517 = call "Fire User Event - Stop.vi"("User Event - Stop"=w1063) -> ("error out"=w1065:errorcluster)  [unwired: 10 in]
        n518 = Release Queue(queue=w1070, error in (no error)=w1064) -> (error out=w1067:errorcluster)  [unwired: 1 in, 2 out]
        n519 = Merge Errors(w1065, w1067) -> (w1066:errorcluster)
      }
      frame Default {
        # "'Default' case only runs if there is a message that isn't defined in any of the other cases.  Output a programming error."
        n520 = xnode "Error Ring"("parameter 0"=w1071) -> ("error out"=w1072:errorcluster)
      }
    }
    n521 = call "LAB-IQ Error Handler - Message Handling Loop.vi"("error in (no error)"=w1019, "Message Queue"=w1021) -> ("dup error in"=w1020:errorcluster)  [unwired: 8 in, 1 out]
  }
  n522 = while {
    shift-right: [w1091] -> _
    shift-left: w6 -> [w1092]
    tunnel: [w1085] -> _
    tunnel: w1 -> [w1083]
    tunnel: w4 -> [w1082]
    tunnel: w5 -> [w1081]
    stop <- w1090 stop-if-true
    # "Report  Handling Loop"
    n523 = call "Dequeue Message.vi"("error in (no error)"=w1082, "Message Queue"=w1083) -> ("error out"=w1089:errorcluster, "Message Data"=w1087:variant, "Message"=w1088:string, "dup Message Queue"=w1086:refnum<queue>)  [unwired: 6 in]
    n524 = case "Message Cases" shown="\"init\"" w1088 {
      selector: w1088 -> [_ _ _ _ _ w1136]
      tunnel: w1086 -> [w1093 w1104 _ w1123 w1135 _]
      tunnel: w1089 -> [w1096 w1101 w1120 w1127 w1129 _]
      tunnel: [w1097 w1105 w1114 w1125 w1131 w1137] -> w1084
      tunnel: w1092 -> [w1095 w1103 w1119 w1126 w1134 w1138]
      tunnel: [w1095 w1103 w1119 w1126 w1134 w1138] -> w1091
      tunnel: [_ _ _ _ TRUE _] -> w1090
      tunnel: w1087 -> [_ _ w1118 _ _ _]
      tunnel: w1081 -> [_ _ _ _ w1128 _]
      frame "init" {
        # "Initialize - All initialization work should take place in this message, since other loops can potentially enqueue messages that execute immediately after this one."
        n525 = call-poly "Enqueue Message.vi"("error in (no error)"=w1096, "Message"="Report Main", "Message Queue"=w1093) -> ("error out"=w1097:errorcluster)  [unwired: 7 in, 1 out]
      }
      frame "Report Main" {
        n526 = Unbundle By Name(w1103) -> ("Main Home Screen.EXIT"=w1102:refnum<vi>)
        n527 = property class="Bool (strict)"(reference=w1102) -> (reference out=w1099:refnum<vi>, error out=w1100:errorcluster, "Value"=w1098:bool)  [unwired: 1 in]
        n528 = case shown="False" w1098 {
          tunnel: [w1108 w1112] -> w1105
          tunnel: w1104 -> [w1107 w1111]
          tunnel: w1101 -> [w1106 w1110]
          frame True {
            n529 = call-poly "Enqueue Message.vi"("error in (no error)"=w1106, "Message"="Confirm Quit", "Message Queue"=w1107) -> ("error out"=w1108:errorcluster)  [unwired: 7 in, 1 out]
          }
          frame False {
            n530 = call-poly "Enqueue Message.vi"("error in (no error)"=w1110, "Message"="Report Main", "Message Queue"=w1111) -> ("error out"=w1112:errorcluster)  [unwired: 7 in, 1 out]
          }
        }
        n531 = Close Reference(reference=w1099, error in (no error)=w1100) -> ()  [unwired: 1 out]
      }
      frame "Error" {
        # "#CodeRecommended - If you ever change the name of this \"Error\" message, you'll need to update the name in the Check Loop Error.vi as well."
        # "#CodeRecommended - Consider creating a system for logging errors in some way. These errors are for notification purposes only. Handling of specific errors should be performed in the message frames that generated the error."
        # "Error - Display an error dialog. This message is sent by the \"Error Handler\" VIs at the end of other loops in this application."
        n532 = Variant To Data(error in=w1120, type=errorcluster {"status"=FALSE, "code"=0, "source"=""} ("error constant"), Variant=w1118) -> (data=w1116:errorcluster, error out=w1115:errorcluster)
        n533 = call <vilib>:"Simple Error Handler.vi"("error in (no error)"=w1116) -> ()  [unwired: 4 in, 5 out]
        n534 = Merge Errors(w1115) -> (w1114:errorcluster)
      }
      frame "Confirm Quit" {
        # "#CodeNeeded - If you want to provide an \"Are you sure\" dialog (or some other notification) before the application exits, place that code here. This message is typically sent from a Panel Close? event."
        # "Confirm Quit - Message that can confirm whether or not the user wants to exit the application."
        n535 = call-poly "Enqueue Message.vi"("Priority Message? (F)"=TRUE, "error in (no error)"=w1127, "Message"="Exit", "Message Queue"=w1123) -> ("error out"=w1124:errorcluster)  [unwired: 6 in, 1 out]
        n536 = Merge Errors(w1124) -> (w1125:errorcluster)
      }
      frame "Exit" {
        # "Stop the VI"
        # "Release the message queue reference"
        # "#CodeNeeded - Add any required cleanup code here. Note that if 'Exit' was called as a result of an error, an error dialog will be displayed. Add any custom error handling for an 'Exit' condition here as well."
        # "Exit - Exit the application."
        n537 = call "Fire User Event - Stop.vi"("User Event - Stop"=w1128) -> ("error out"=w1130:errorcluster)  [unwired: 10 in]
        n538 = Release Queue(queue=w1135, error in (no error)=w1129) -> (error out=w1132:errorcluster)  [unwired: 1 in, 2 out]
        n539 = Merge Errors(w1130, w1132) -> (w1131:errorcluster)
      }
      frame Default {
        # "'Default' case only runs if there is a message that isn't defined in any of the other cases.  Output a programming error."
        n540 = xnode "Error Ring"("parameter 0"=w1136) -> ("error out"=w1137:errorcluster)
      }
    }
    n541 = call "LAB-IQ Error Handler - Message Handling Loop.vi"("error in (no error)"=w1084, "Message Queue"=w1086) -> ("dup error in"=w1085:errorcluster)  [unwired: 8 in, 1 out]
  }
  n542 = Unregister For Events(event registration refnum=w42, error in=w40) -> (error out=w43:errorcluster)
  n543 = Merge Errors(w43, w46, w18, w15, w12, w11) -> (w44:errorcluster)
  n544 = call "Destroy User Event - Stop.vi"("error in (no error)"=w44, "User Event - Stop"=w5) -> ("error out"=w41:errorcluster)  [unwired: 9 in]
  n545 = disable-structure shown="RUN_TIME_ENGINE==True" {
    disable-tunnel: w41 -> [_ _]
    frame condition #0 (active) {
    }
    frame condition #1 {
      # "Call Quit LabVIEW if running as a built application."
      n546 = Quit LabVIEW() -> ()  [unwired: 1 in]
    }
  }
